vi "Live Capture Functional Stack4.64bit.vi"() -> ()   [LabVIEW 2014]
uses:
  subvis/Stack Track.ctl
  subvis/Stack_State.ctl
  Desktop/camtiff/ctiff.llb/__CTIFFNewFileAndStyleUINT16.vi
  Desktop/camtiff/ctiff.llb/__CTIFFAddNewPageUINT16.vi
  CameraControlTypeDef.ctl
panel:
  out "Image 2":u16[][](graph) caption="Image"
  in  "Slit Width / Lines 2":sgl=150.0
  out "Frame Index":i32
  in  "Temp":path=path "C:/temp.tmp"
  in  "Frames":i32=100
  in  "HardDisk Record":bool
  in  "Internal Line Interval":dbl
  in  "Slit Width / Lines":sgl=150.0
  in  "Camera Readout Mode":u16(ring)=12 items=["Full Frame"=1, "Slit Scanning"=12]
  in  "Readout Direction":sgl(ring)=1.0 items=["Forward"=1, "Backward"=2]
  in  "Trigger Mode":sgl(ring)=1.0 items=["Normal"=1, "Start "=6]
  in  "Trigger Source":sgl(ring)=2.0 items=["Internal"=1, "External"=2]
  out "State":T1=enum."Start Sequence"
  out "Image":u16[][](graph)
  out "Saving":bool
  in  "AutoIncrement":bool=TRUE
  in  "Path":path=path "C:/Users/spim/Desktop/Craig Cap/temp/a.tiff"
  in  "Frames":i32=100
  out "Frame Index":i32
  out "error out":errorcluster
  in  "stop":bool
  in  "Ram Record":bool
  out "Total Frames":i32
  out "Elapsed Time":u32
  out "Software FPS":dbl
  out "Camera FPS":dbl
  in  "H Offset":i32 min=0 max=0
  in  "H Width":i32 min=0 max=0
  out "SMD":dbl
  out "SHO":i32
  in  "V Offset":i32 min=0 max=0
  in  "V Width":i32 min=0 max=0
  in  "Binning":u16(ring) items=["1x1"=1, "2x2"=2, "4x4"=4]
  out "SHW":i32
  out "SVO":i32
  out "SVW":i32
  in  "Scan Mode":dbl min=0.0 max=0.0
  in  "Exposure":dbl min=0.0 max=0.0
  out "EXP":dbl
  out "Camera Model":string
  out "Camera Version":string
  out "Camera Serial":string
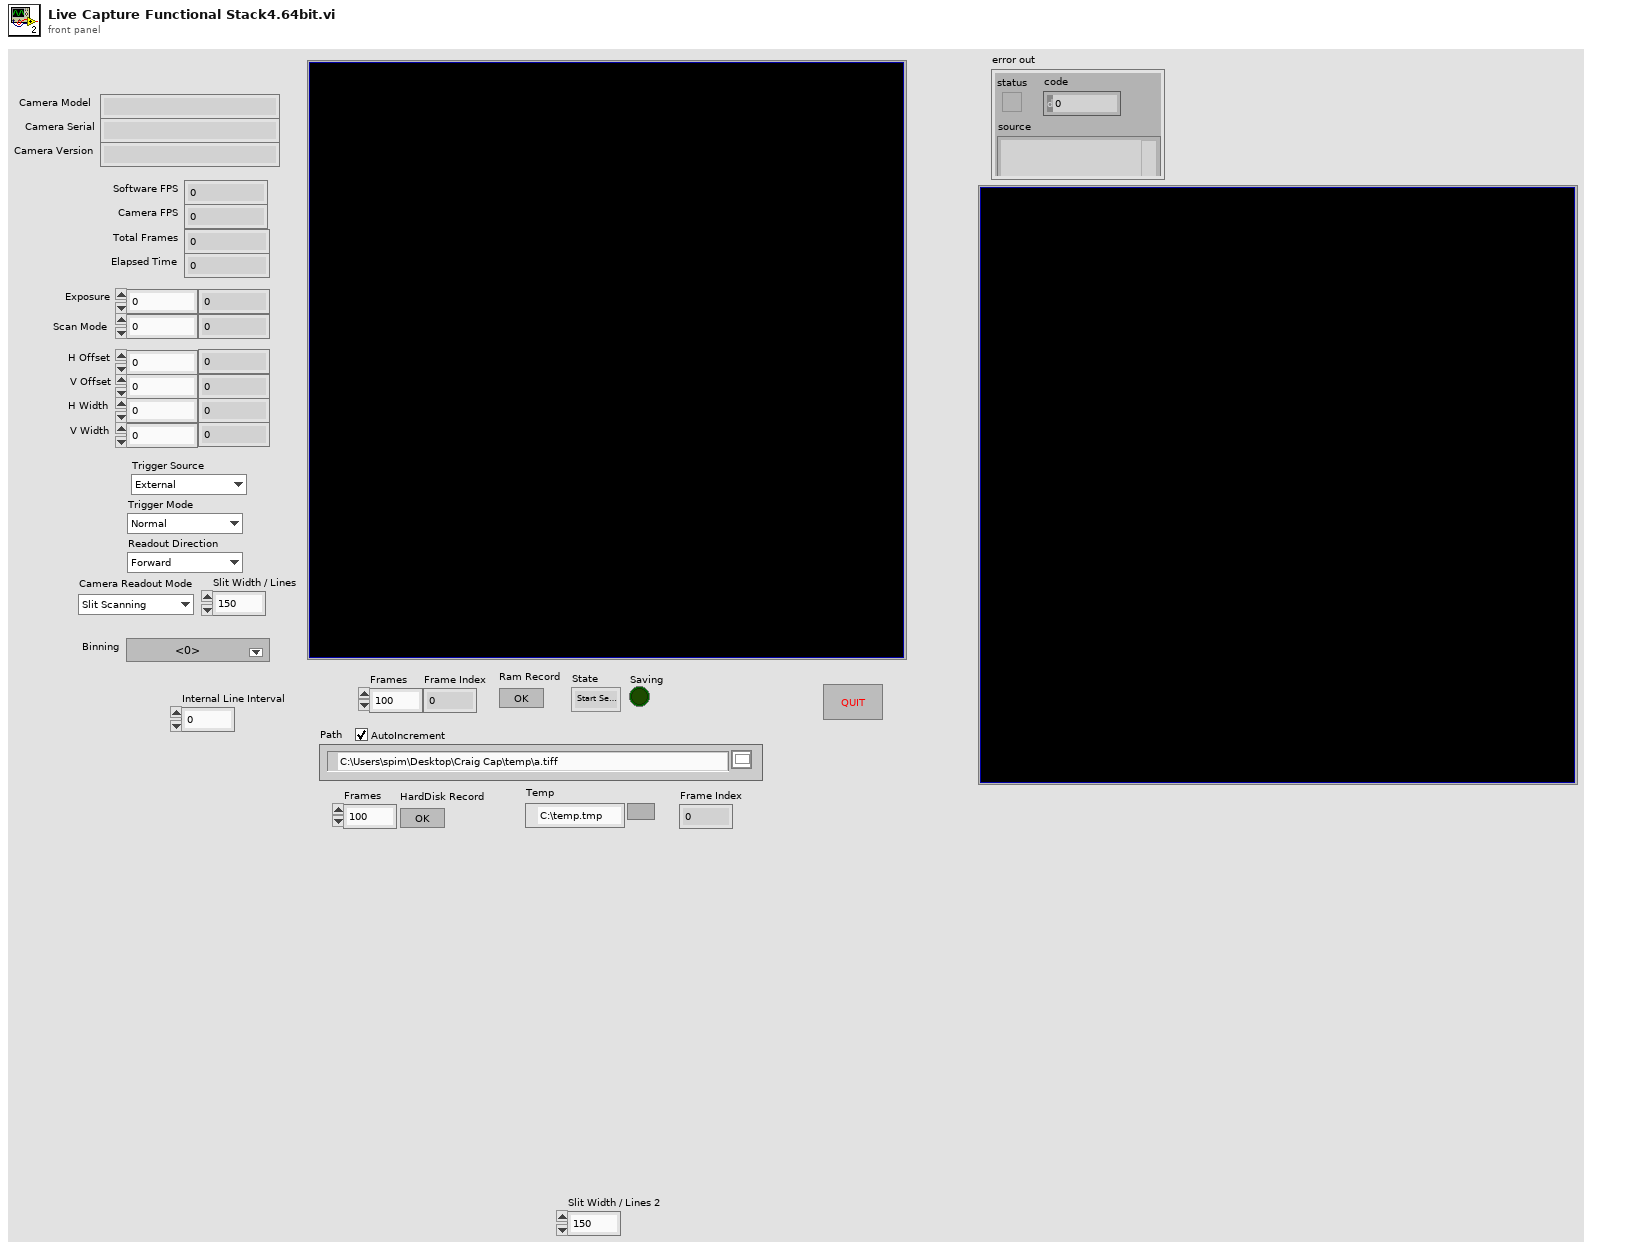
[diagram p1: front panel]
types:
  T1 = typedef "Stack Track.ctl" = enum16{"Idle", "Start Sequence", "Read Disk", "STOP", "Collecting", "End"}
  T2 = typedef "Stack_State.ctl" = cluster{"State":T1, "Stack Number":i32, "Image":u16[][]}
  T3 = typedef "CameraControlTypeDef.ctl" = enum16{"Ram Record", "HardDisk Record", "Disengage Update", "Update", "Idle"}
  T4 = enum8{"Enabled", "Disabled", "Disabled and Grayed Out"}
  T5 = cluster{"Model":string, "Camera ID":string, "Firmware":string}
  T6 = cluster{"Value":i32, "Minimum":i32, "Maximum":i32, "Increment":i32}
  T7 = cluster{"height":u32, "width":u32, "datatype":u32}
  T8 = cluster{"H Offset":i32, "V Offset":i32, "H Width":i32, "V Width":i32}
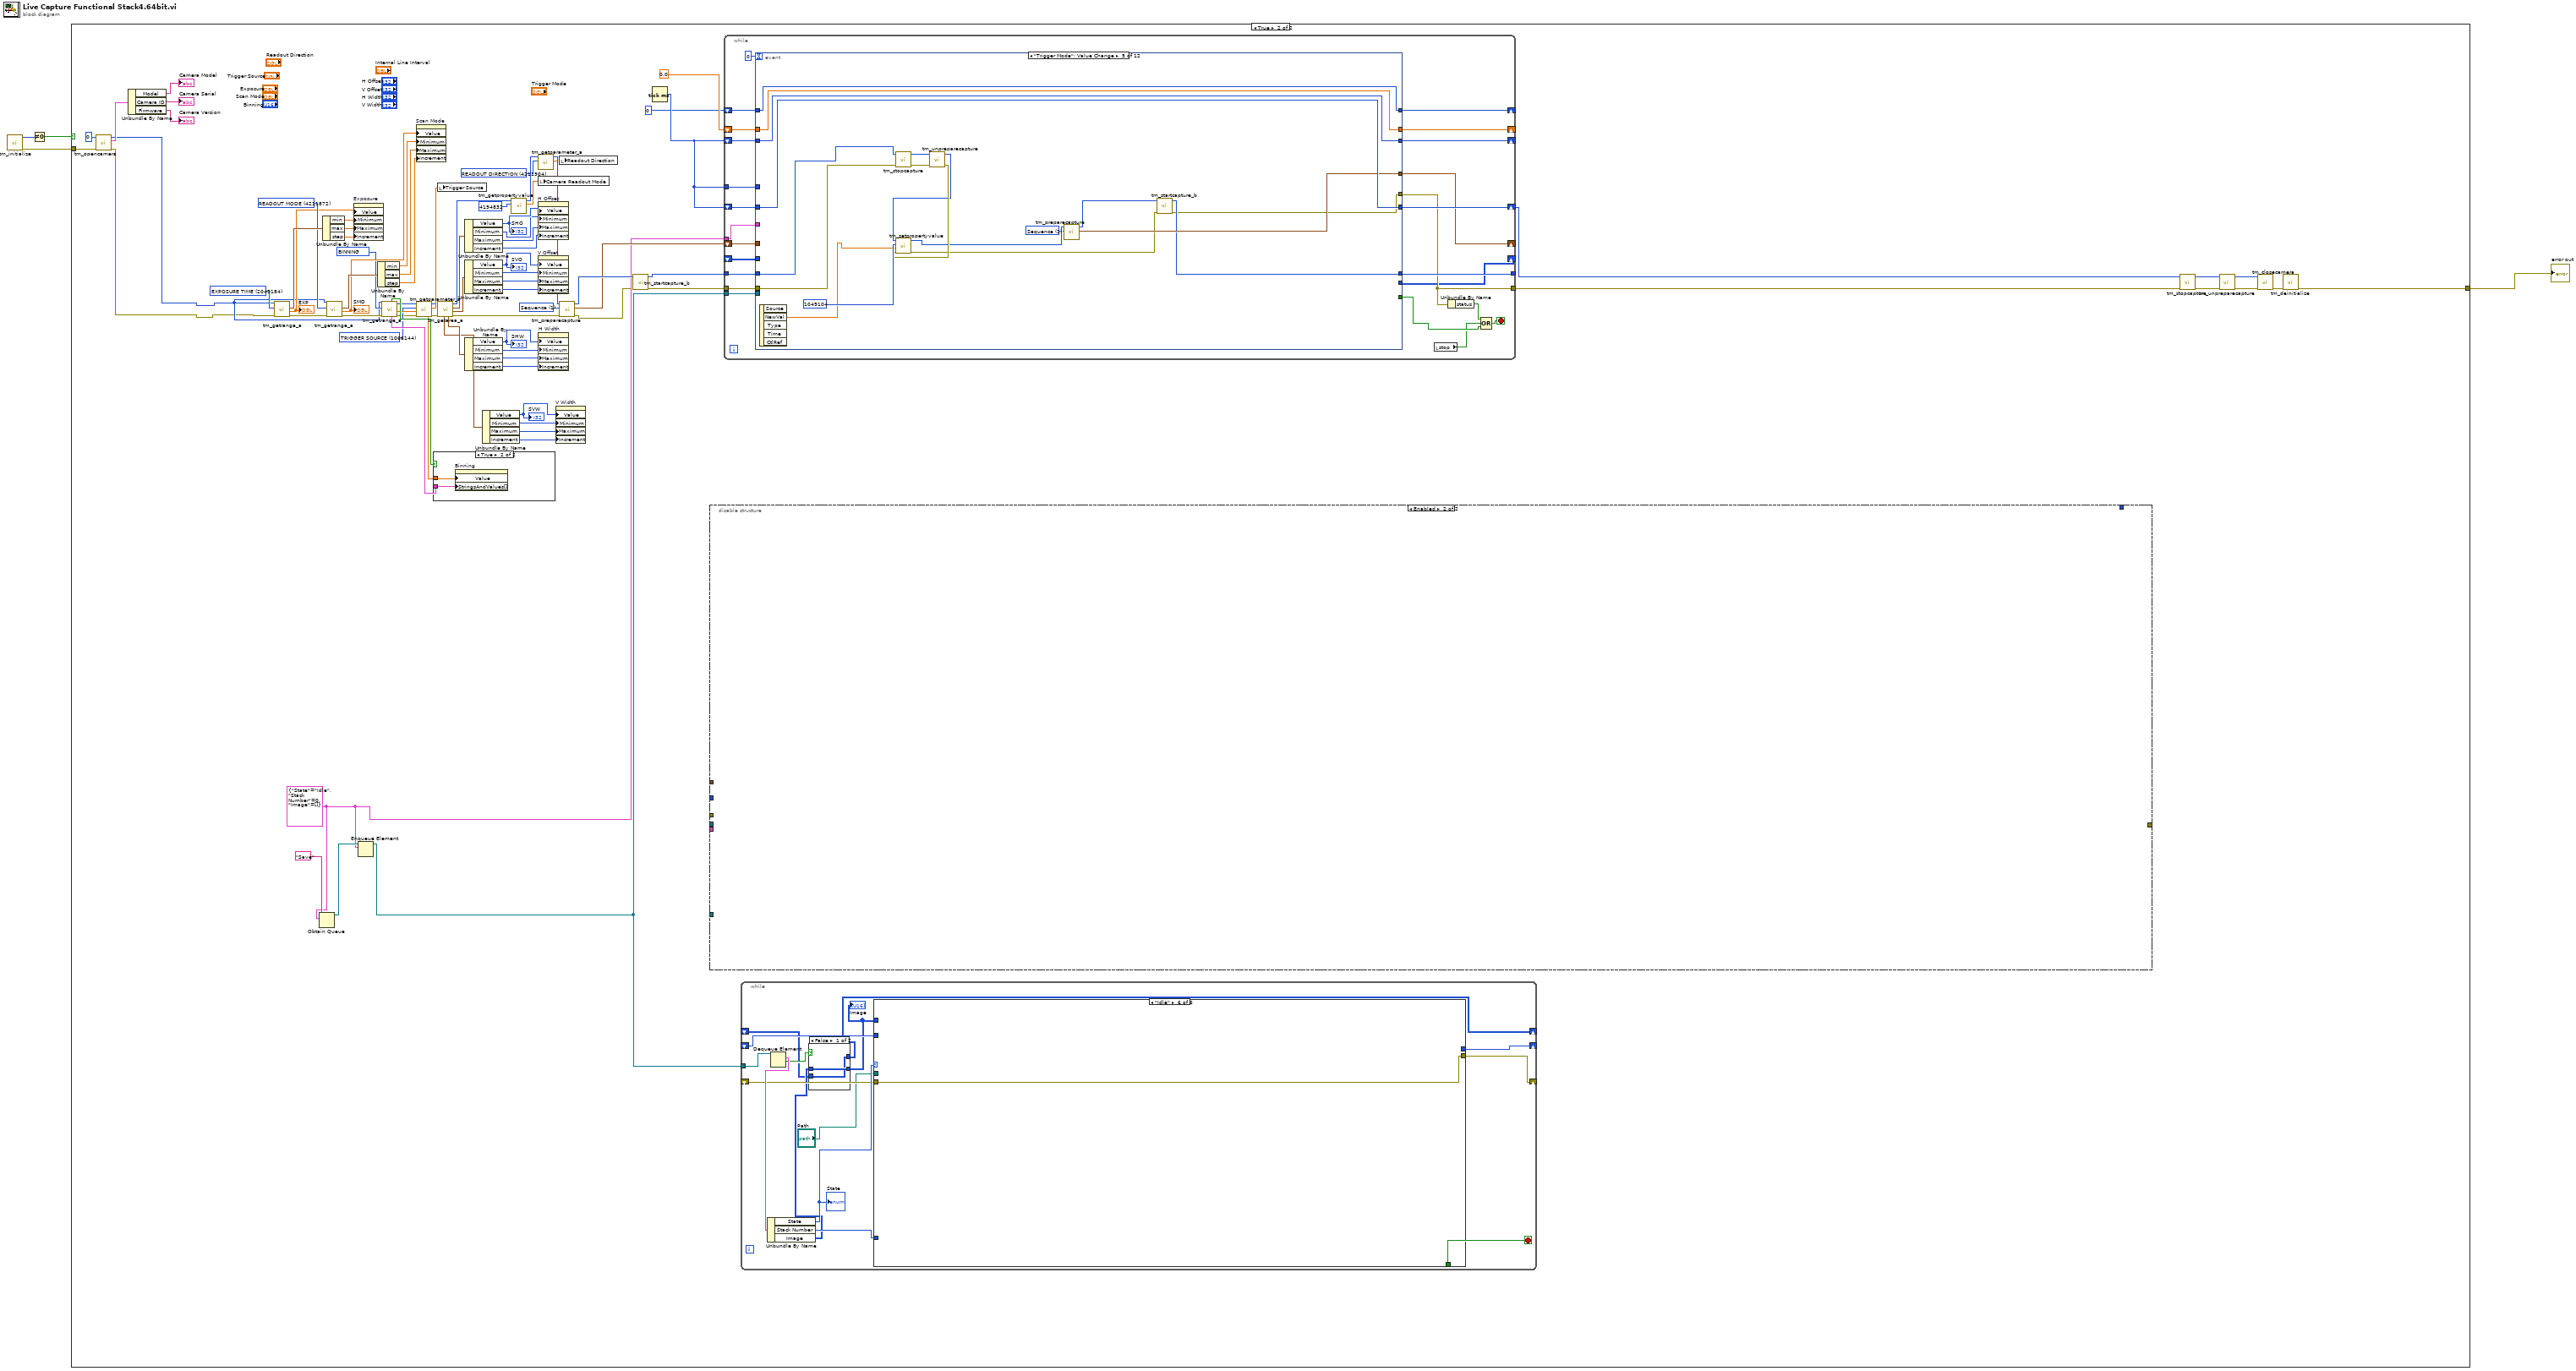
[diagram p0: block diagram]
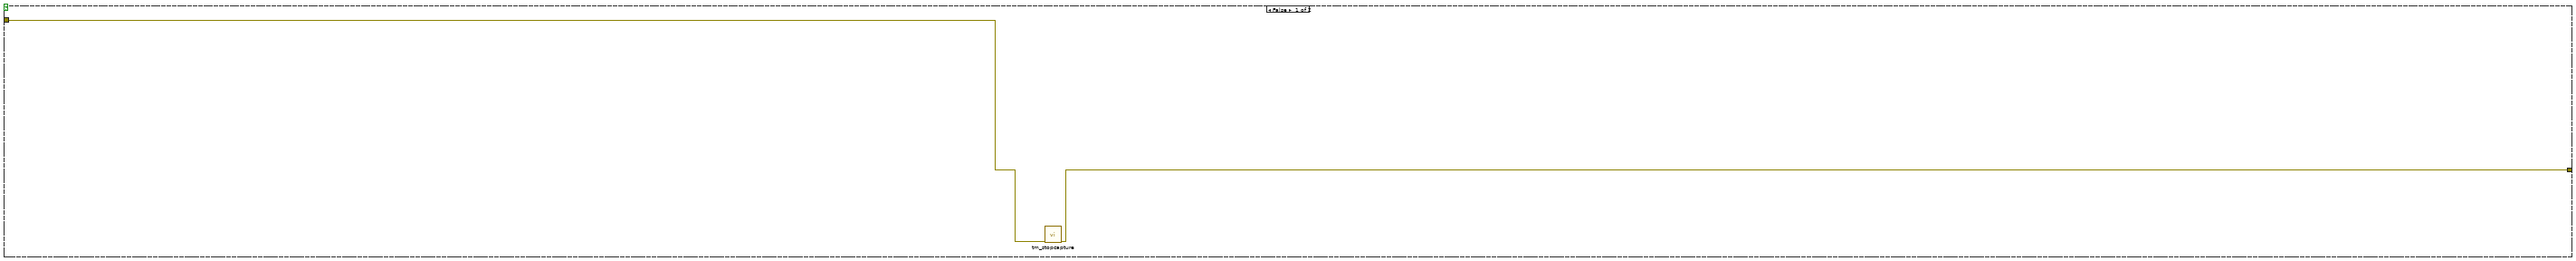
[diagram p2: hidden frame]
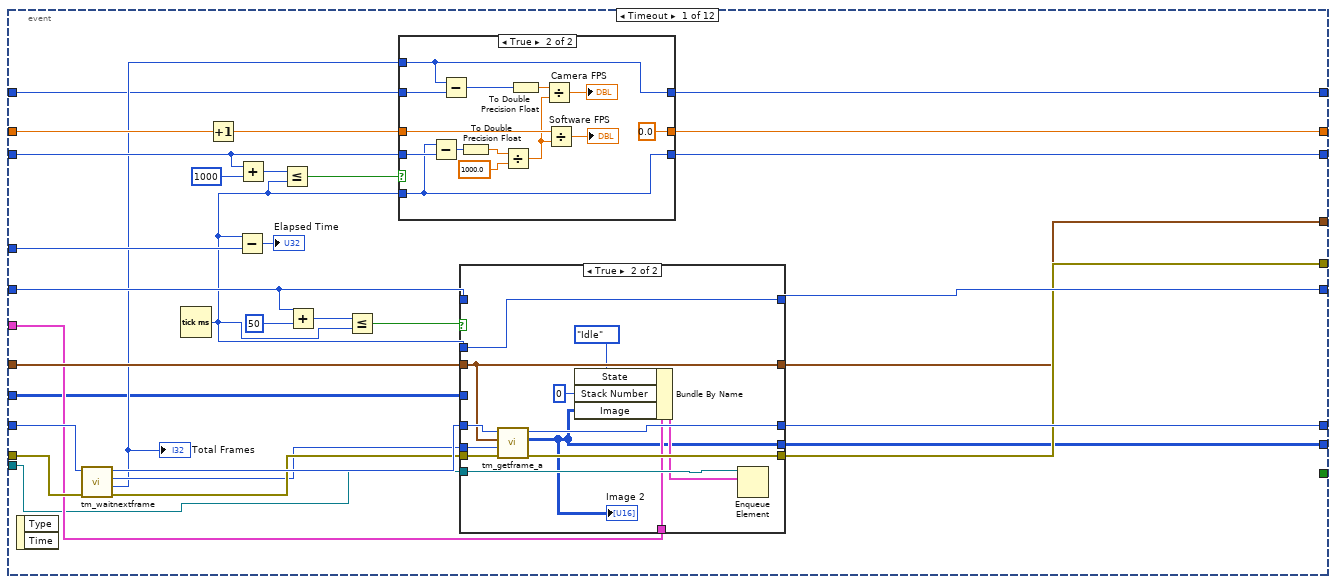
[diagram p3: hidden frame]
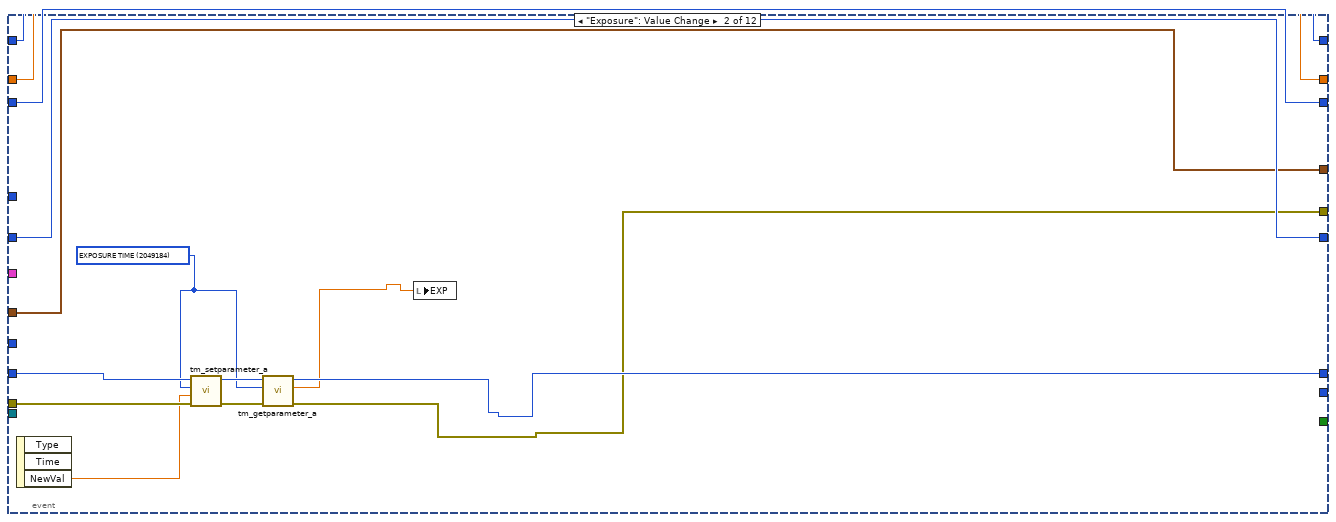
[diagram p6: hidden frame]
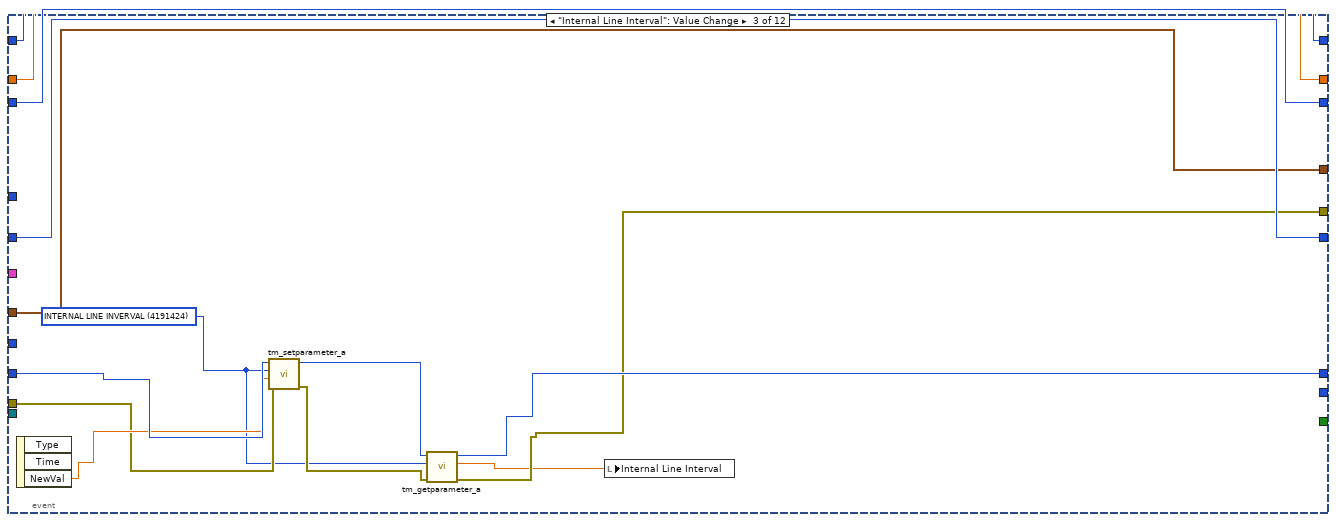
[diagram p7: hidden frame]
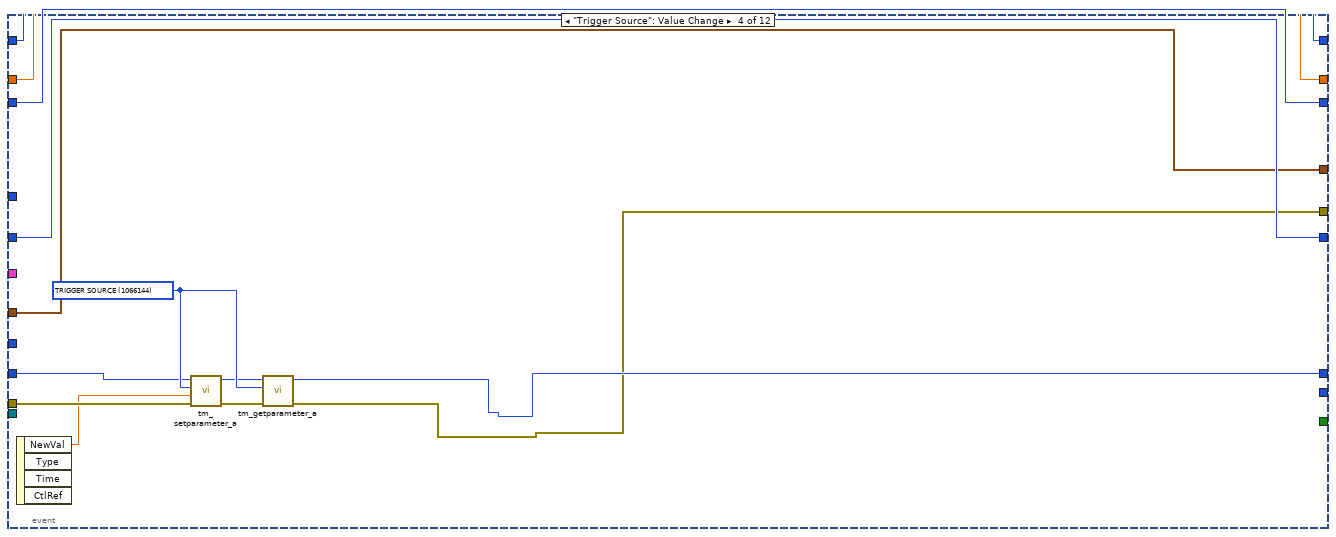
[diagram p8: hidden frame]
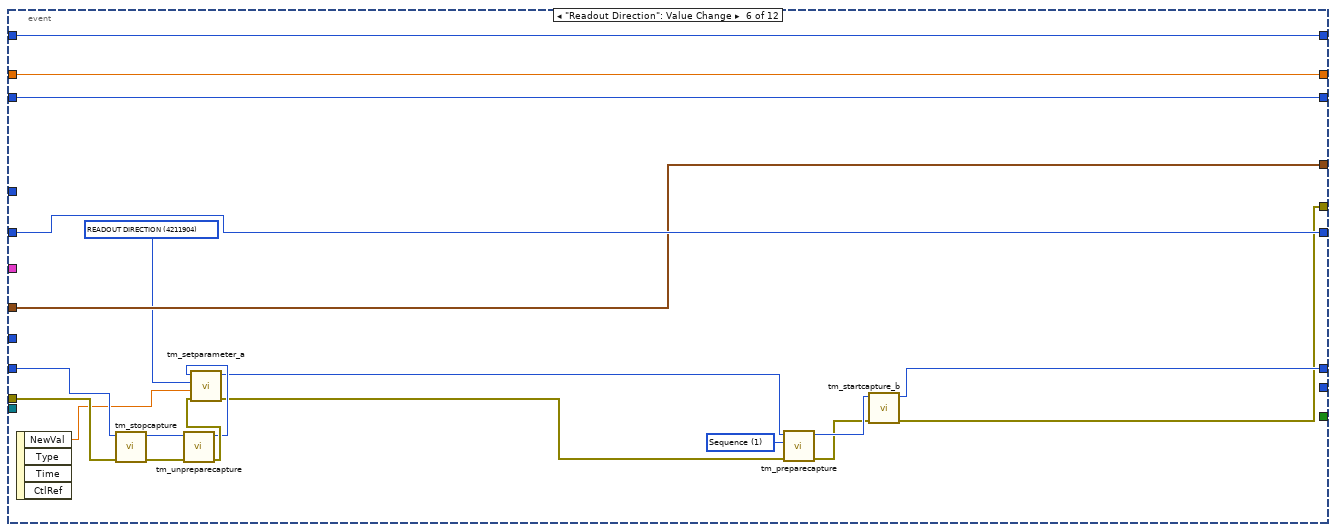
[diagram p9: hidden frame]
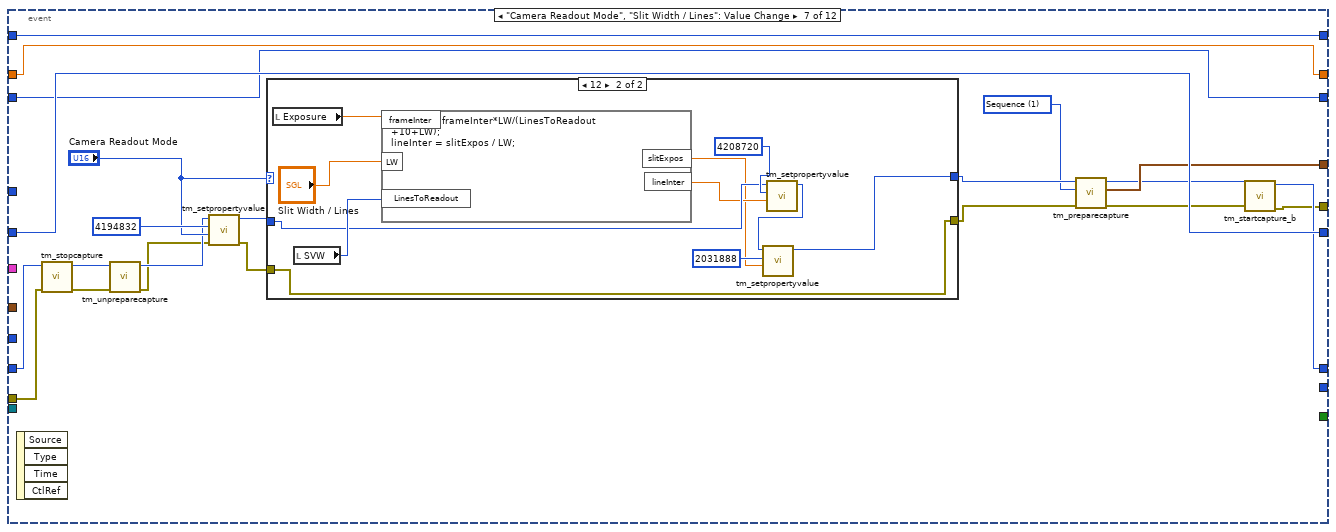
[diagram p10: hidden frame]
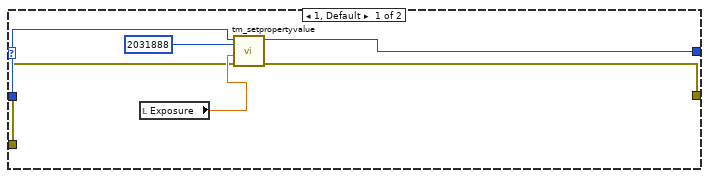
[diagram p11: hidden frame]
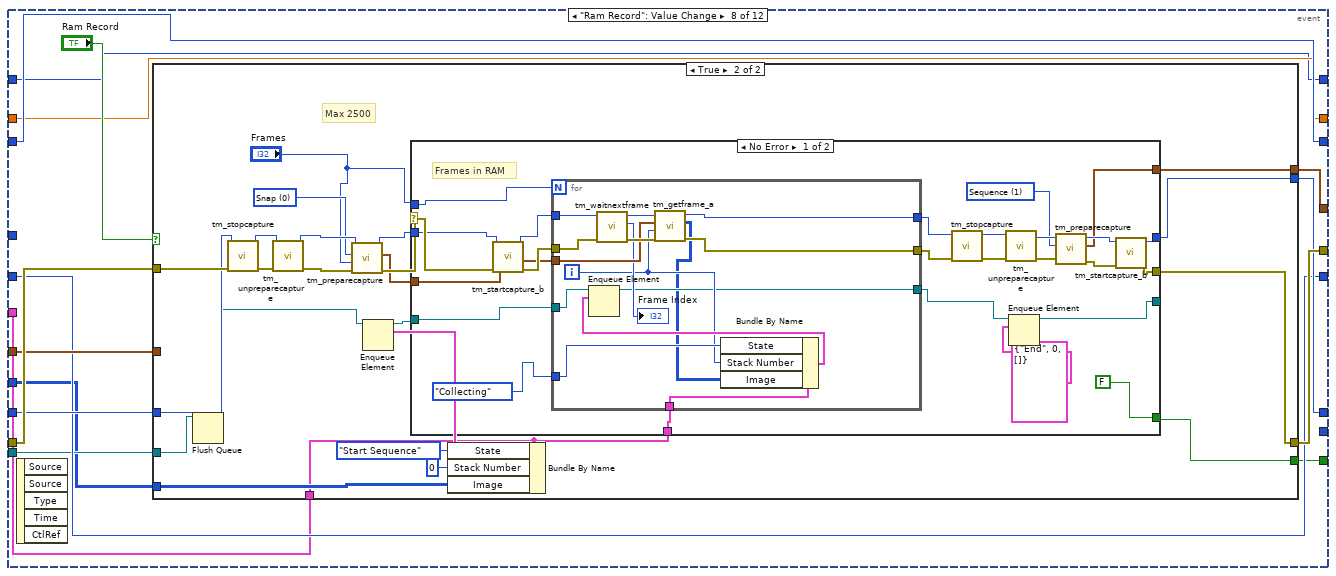
[diagram p12: hidden frame]
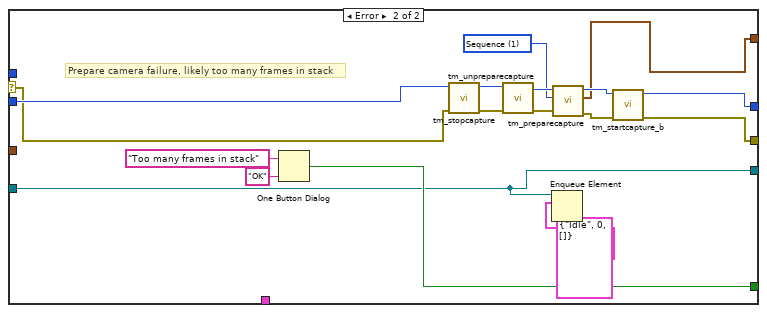
[diagram p14: hidden frame]
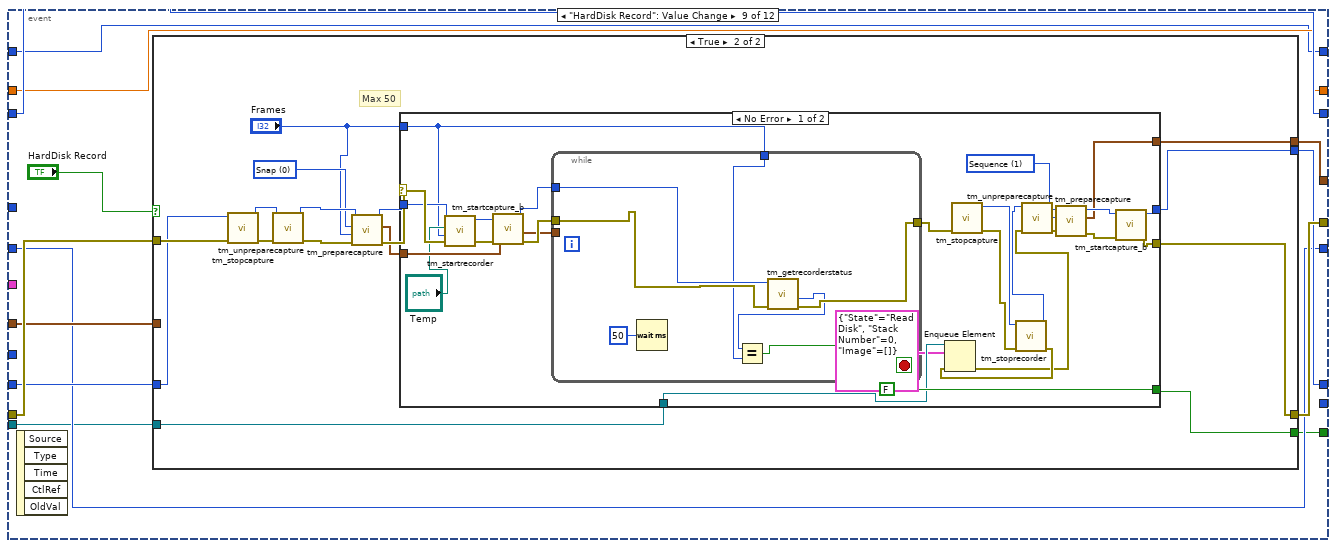
[diagram p15: hidden frame]
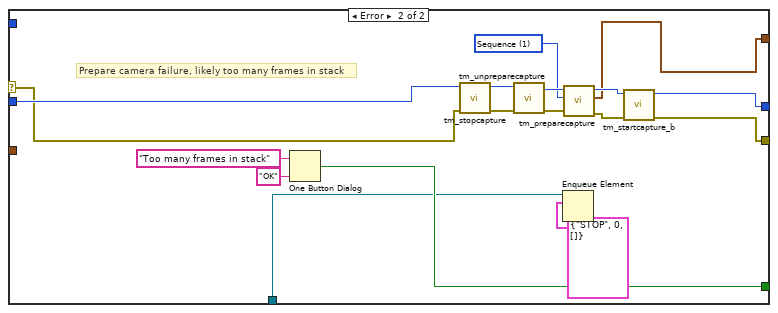
[diagram p17: hidden frame]
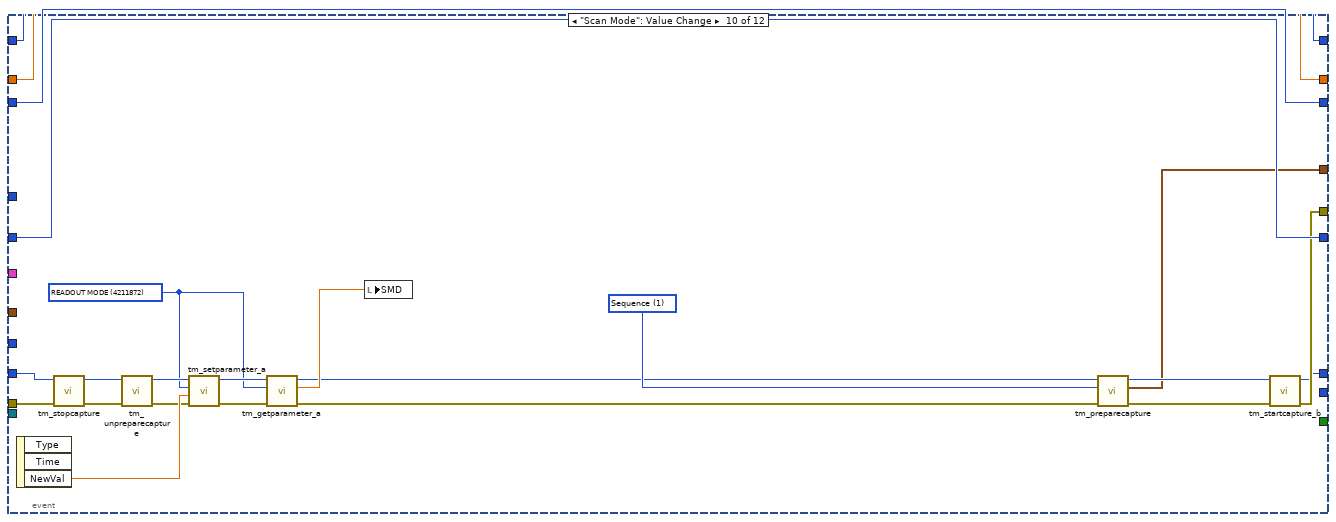
[diagram p18: hidden frame]
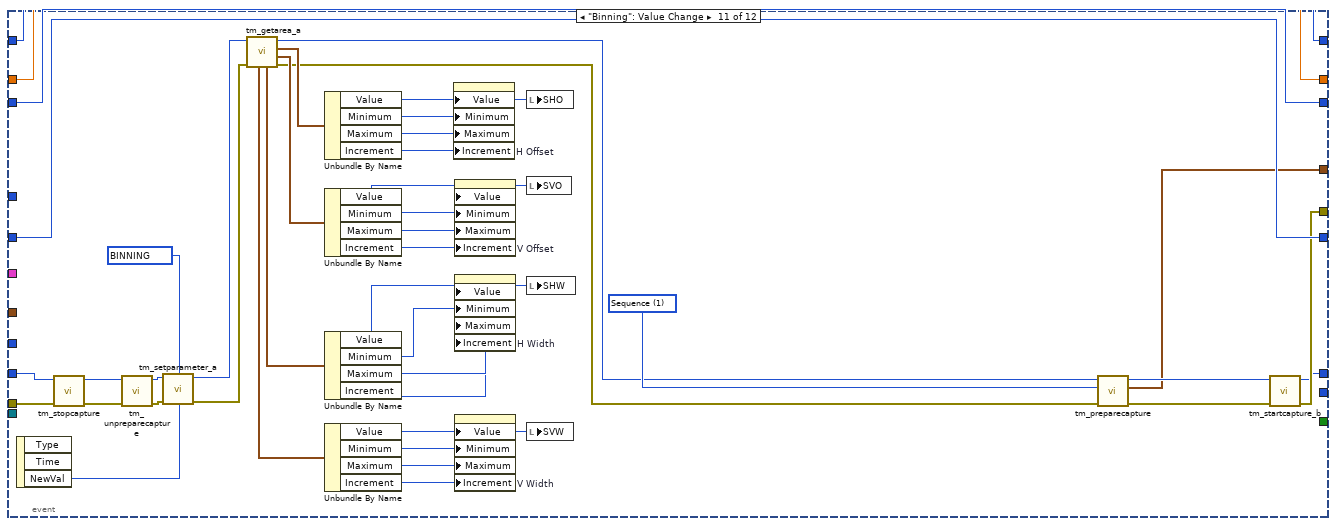
[diagram p19: hidden frame]
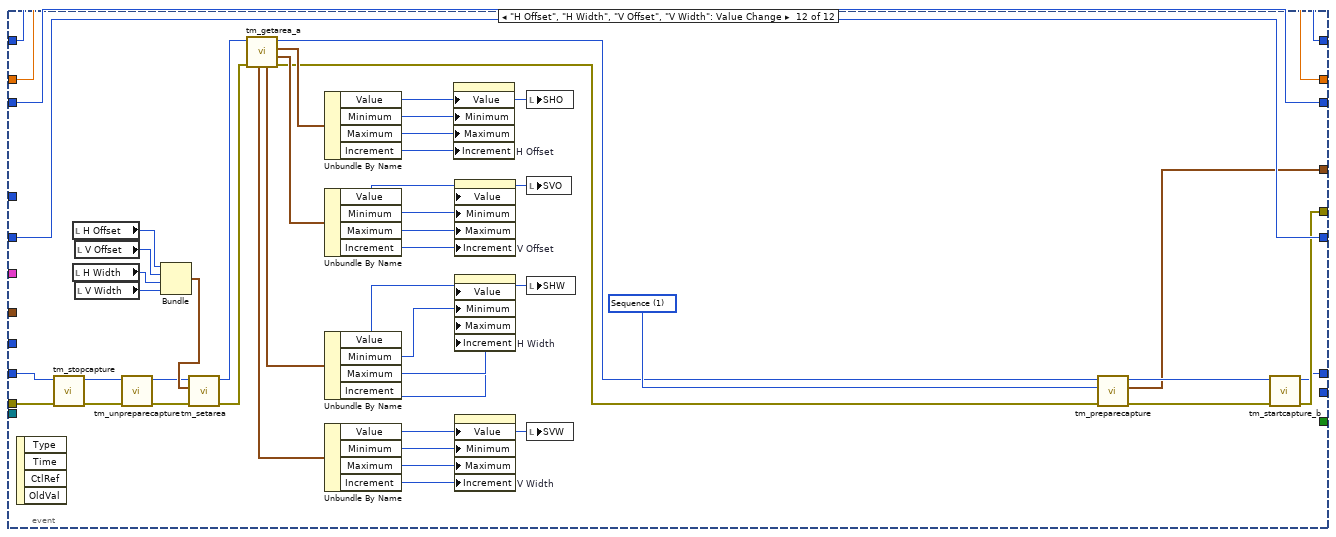
[diagram p20: hidden frame]
diagram:
  n1 = call <userlib>:"tm_initialize.vi"() -> ("error out"=w2:errorcluster, "Number Of Cameras"=w1:u32)  [unwired: 8 in, 2 out]
  n2 = Not Equal To 0?(x=w1) -> (x != 0?=w4:bool)
  n3 = case shown="True" w4 {
    tunnel: [w5 w84] -> w3
    tunnel: w2 -> [w6 w87]
    frame False {
      n4 = call <userlib>:"tm_stopcapture.vi"("error in (no error)"=w6) -> ("error out"=w5:errorcluster)  [unwired: 9 in, 1 out]
    }
    frame True {
      w19 = u32 4211904 items=["SENSOR MODE"=4212128, "CCD MODE"=4212384, "READOUT MODE"=4211872, "ACTIVE VIEW INDEX"=4343136, "BITS PER CHANNEL"=4342976, "IMAGE PIXEL TYPE"=4343296, "BINNING"=4215968, "EXPOSURE TIME"=2049184, "CONTRAST GAIN"=3163312, "CONTRAST OFFSET"=3163328, "LIGHT MODE"=2114720, "SENSITIVITY"=2114992, "PHOTON IMAGING MODE"=2115200, "HIGH DYNAMIC RANGE MODE"=3163360, "WHITE BALANCE"=3163568, "TEMPERATURE"=2115232, "TEMPERATURE TARGET"=2115264, "SENSOR COOLER FAN"=2115296, "LINEBUNDLE HEIGHT"=4212192, "MECHANICAL SHUTTER"=2115488, "BACK FOCUS POSITION"=8422304, "TRIGGER CONNECTOR"=1066432, "TRIGGER SOURCE"=1066144, "OUTPUT TRIGGER SOURCE"=1852576, "TRIGGER GLOBAL EXPOSURE"=2049680, "FIRST TRIGGER BEHAVIOR"=2049696, "CHANNEL SYNC"=1852352, "READOUT DIRECTION"=4211904, "PRE HSYNC COUNT"=1852704] ("Parameter")
      w29 = u32 1066144 items=["SENSOR MODE"=4212128, "CCD MODE"=4212384, "READOUT MODE"=4211872, "ACTIVE VIEW INDEX"=4343136, "BITS PER CHANNEL"=4342976, "IMAGE PIXEL TYPE"=4343296, "BINNING"=4215968, "EXPOSURE TIME"=2049184, "CONTRAST GAIN"=3163312, "CONTRAST OFFSET"=3163328, "LIGHT MODE"=2114720, "SENSITIVITY"=2114992, "PHOTON IMAGING MODE"=2115200, "HIGH DYNAMIC RANGE MODE"=3163360, "WHITE BALANCE"=3163568, "TEMPERATURE"=2115232, "TEMPERATURE TARGET"=2115264, "SENSOR COOLER FAN"=2115296, "LINEBUNDLE HEIGHT"=4212192, "MECHANICAL SHUTTER"=2115488, "BACK FOCUS POSITION"=8422304, "TRIGGER CONNECTOR"=1066432, "TRIGGER SOURCE"=1066144, "OUTPUT TRIGGER SOURCE"=1852576, "TRIGGER GLOBAL EXPOSURE"=2049680, "FIRST TRIGGER BEHAVIOR"=2049696, "CHANNEL SYNC"=1852352, "READOUT DIRECTION"=4211904, "PRE HSYNC COUNT"=1852704] ("Parameter")
      w12 = T2 {"State"=enum."Idle", "Stack Number"=0, "Image"=[]} ("input cluster")
      w34 = u32 2049184 items=["BINNING"=4215968, "BITS PER CHANNEL"=4342976, "ACTIVE VIEW INDEX"=4343136, "CCD MODE"=4212384, "SENSOR MODE"=4212128, "READOUT MODE"=4211872, "EXPOSURE TIME"=2049184, "CONTRAST GAIN"=3163312, "CONTRAST OFFSET"=3163328, "LIGHT MODE"=2114720, "SENSITIVITY"=2114992, "WHITE BALANCE"=3163568, "PHOTON IMAGING MODE"=2115200, "HIGH DYNAMIC RANGE MODE"=3163360, "TRIGGER SOURCE"=1066144, "TRIGGER ACTIVE"=1066160, "TRIGGER MODE"=1066400, "TRIGGER POLARITY"=1066416, "TRIGGER GLOBAL EXPOSURE"=2049680, "FIRST TRIGGER BEHAVIOR"=2049696, "TRIGGER TIMES"=1066448, "OUTPUT TRIGGER POLARITY"=1852592, "OUTPUT TRIGGER DELAY"=1852624, "OUTPUT TRIGGER PERIOD"=1852640, "TEMPERATURE"=2115232, "TEMPERATURE TARGET"=2115264, "SENSOR COOLER FAN"=2115296, "MECHANICAL SHUTTER"=2115488, "BACK FOCUS POSITION"=8422304, "FRAMEBUNDLE MODE"=4346784, "FRAMEBUNDLE NUMBER"=4346800, "LINEBUNDLE HEIGHT"=4212192, "TRIGGER CONNECTOR"=1066432, "IMAGE PIXEL TYPE"=4343296, "OUTPUT TRIGGER KIND"=1852656, "READOUT DIRECTION"=4211904, "CHANNEL SYNC"=1852352] ("Parameter")
      w35 = u32 4211872 items=["BINNING"=4215968, "BITS PER CHANNEL"=4342976, "ACTIVE VIEW INDEX"=4343136, "CCD MODE"=4212384, "SENSOR MODE"=4212128, "READOUT MODE"=4211872, "EXPOSURE TIME"=2049184, "CONTRAST GAIN"=3163312, "CONTRAST OFFSET"=3163328, "LIGHT MODE"=2114720, "SENSITIVITY"=2114992, "WHITE BALANCE"=3163568, "PHOTON IMAGING MODE"=2115200, "HIGH DYNAMIC RANGE MODE"=3163360, "TRIGGER SOURCE"=1066144, "TRIGGER ACTIVE"=1066160, "TRIGGER MODE"=1066400, "TRIGGER POLARITY"=1066416, "TRIGGER GLOBAL EXPOSURE"=2049680, "FIRST TRIGGER BEHAVIOR"=2049696, "TRIGGER TIMES"=1066448, "OUTPUT TRIGGER POLARITY"=1852592, "OUTPUT TRIGGER DELAY"=1852624, "OUTPUT TRIGGER PERIOD"=1852640, "TEMPERATURE"=2115232, "TEMPERATURE TARGET"=2115264, "SENSOR COOLER FAN"=2115296, "MECHANICAL SHUTTER"=2115488, "BACK FOCUS POSITION"=8422304, "FRAMEBUNDLE MODE"=4346784, "FRAMEBUNDLE NUMBER"=4346800, "LINEBUNDLE HEIGHT"=4212192, "TRIGGER CONNECTOR"=1066432, "IMAGE PIXEL TYPE"=4343296, "OUTPUT TRIGGER KIND"=1852656, "READOUT DIRECTION"=4211904, "CHANNEL SYNC"=1852352] ("Parameter")
      w36 = u32 4215968 items=["BINNING"=4215968, "BITS PER CHANNEL"=4342976, "ACTIVE VIEW INDEX"=4343136, "CCD MODE"=4212384, "SENSOR MODE"=4212128, "READOUT MODE"=4211872, "EXPOSURE TIME"=2049184, "CONTRAST GAIN"=3163312, "CONTRAST OFFSET"=3163328, "LIGHT MODE"=2114720, "SENSITIVITY"=2114992, "WHITE BALANCE"=3163568, "PHOTON IMAGING MODE"=2115200, "HIGH DYNAMIC RANGE MODE"=3163360, "TRIGGER SOURCE"=1066144, "TRIGGER ACTIVE"=1066160, "TRIGGER MODE"=1066400, "TRIGGER POLARITY"=1066416, "TRIGGER GLOBAL EXPOSURE"=2049680, "FIRST TRIGGER BEHAVIOR"=2049696, "TRIGGER TIMES"=1066448, "OUTPUT TRIGGER POLARITY"=1852592, "OUTPUT TRIGGER DELAY"=1852624, "OUTPUT TRIGGER PERIOD"=1852640, "TEMPERATURE"=2115232, "TEMPERATURE TARGET"=2115264, "SENSOR COOLER FAN"=2115296, "MECHANICAL SHUTTER"=2115488, "BACK FOCUS POSITION"=8422304, "FRAMEBUNDLE MODE"=4346784, "FRAMEBUNDLE NUMBER"=4346800, "LINEBUNDLE HEIGHT"=4212192, "TRIGGER CONNECTOR"=1066432, "IMAGE PIXEL TYPE"=4343296, "OUTPUT TRIGGER KIND"=1852656, "READOUT DIRECTION"=4211904, "CHANNEL SYNC"=1852352] ("Parameter")
      w82 = 1 items=["Snap", "Sequence"] ("Capture mode")
      n5 = call <userlib>:"tm_opencamera.vi"("error in (no error)"=w87, "Camera Index"=u32 0) -> ("error out"=w7:errorcluster, "Camera Details"=w48:T5, "Handle out"=w8:u32)  [unwired: 7 in]
      n6 = Unbundle By Name(w48) -> ("Model"=→"Camera Model":string, "Camera ID"=→"Camera Serial":string, "Firmware"=→"Camera Version":string)
      n7 = call <userlib>:"tm_getrange_a.vi"("error in (no error)"=w7, "Parameter"=w34, "Handle in"=w8) -> ("error out"=w43:errorcluster, "default"=w32:dbl, "Range"=w44:cluster{"min":dbl, "max":dbl, "step":dbl})  [unwired: 2 in, 4 out]
      "EXP" <- w32
      n8 = Obtain Queue(name (unnamed)="Save", element data type=w12) -> (queue out=w16:refnum<queue>)  [unwired: 3 in, 2 out]
      n9 = Unbundle By Name(w44) -> ("min"=w79:dbl, "max"=w78:dbl, "step"=w77:dbl)
      n10 = call <userlib>:"tm_getrange_a.vi"("error in (no error)"=w43, "Parameter"=w35, "Handle in"=w8) -> ("error out"=w40:errorcluster, "default"=w41:dbl, "Range"=w42:cluster{"min":dbl, "max":dbl, "step":dbl})  [unwired: 2 in, 4 out]
      "SMD" <- w41
      n11 = property on="Exposure" class="DigNum (strict)"("Value"=w32, "Minimum"=w79, "Maximum"=w78, "Increment"=w77) -> ()  [unwired: 2 in, 2 out]
      n12 = Enqueue Element(queue=w16, element=w12) -> (queue out=w15:refnum<queue>)  [unwired: 2 in, 2 out]
      n13 = Unbundle By Name(w42) -> ("min"=w76:dbl, "max"=w75:dbl, "step"=w74:dbl)
      n14 = call <userlib>:"tm_getrange_a.vi"("error in (no error)"=w40, "Parameter"=w36, "Handle in"=w8) -> ("error out"=w26:errorcluster, "default"=w38:dbl, "Handle out"=w28:u32, "Value Names"=w37:cluster{"Name":string, "Value":dbl}[], "Writable"=w39:bool)  [unwired: 2 in, 2 out]
      n15 = property on="Scan Mode" class="DigNum (strict)"("Value"=w41, "Minimum"=w76, "Maximum"=w75, "Increment"=w74) -> ()  [unwired: 2 in, 2 out]
      n16 = call <userlib>:"tm_getparameter_a.vi"("error in (no error)"=w26, "Parameter"=w29, "Handle in"=w28) -> ("error out"=w25:errorcluster, "Value out"=w30:dbl, "Handle out"=w27:u32)  [unwired: 6 in]
      n17 = case shown="True" w39 {
        tunnel: w37 -> [_ w833]
        tunnel: w38 -> [_ w832]
        frame False {
        }
        frame True {
          n18 = property on="Binning" class="Ring (strict)"("Value"=w832, "StringsAndValues[]"=w833) -> ()  [unwired: 2 in, 2 out]
        }
      }
      n19 = local write "Trigger Source"(w30) -> ()
      n20 = call <userlib>:"tm_getarea_a.vi"("error in (no error)"=w25, "Handle in"=w27) -> ("error out"=w31:errorcluster, "V Offset"=w73:T6, "H Offset"=w54:T6, "Handle out"=w22:u32, "H Width"=w72:T6, "V Width"=w71:T6)  [unwired: 4 in]
      n21 = Unbundle By Name(w54) -> ("Value"=w53:i32, "Minimum"=w52:i32, "Maximum"=w51:i32, "Increment"=w50:i32)
      "SHO" <- w53
      n22 = Unbundle By Name(w73) -> ("Value"=w61:i32, "Minimum"=w70:i32, "Maximum"=w69:i32, "Increment"=w68:i32)
      "SVO" <- w61
      n23 = Unbundle By Name(w72) -> ("Value"=w60:i32, "Minimum"=w67:i32, "Maximum"=w66:i32, "Increment"=w65:i32)
      "SHW" <- w60
      n24 = Unbundle By Name(w71) -> ("Value"=w59:i32, "Minimum"=w64:i32, "Maximum"=w63:i32, "Increment"=w62:i32)
      "SVW" <- w59
      n25 = call <userlib>:"tm_getpropertyvalue.vi"("Property ID"=u32 4194832, "Handle in"=w22) -> ("Value in"=w23:sgl, "Handle out"=w21:u32)  [unwired: 7 in, 1 out]
      n26 = call <userlib>:"tm_getparameter_a.vi"("Parameter"=w19, "Handle in"=w21) -> ("Value out"=w18:dbl, "Handle out"=w20:u32)  [unwired: 7 in, 1 out]
      n27 = local write "Camera Readout Mode"(w23) -> ()
      n28 = property on="H Offset" class="DigNum (strict)"("Value"=w53, "Minimum"=w52, "Maximum"=w51, "Increment"=w50) -> ()  [unwired: 2 in, 2 out]
      n29 = property on="V Offset" class="DigNum (strict)"("Value"=w61, "Minimum"=w70, "Maximum"=w69, "Increment"=w68) -> ()  [unwired: 2 in, 2 out]
      n30 = property on="H Width" class="DigNum (strict)"("Value"=w60, "Minimum"=w67, "Maximum"=w66, "Increment"=w65) -> ()  [unwired: 2 in, 2 out]
      n31 = property on="V Width" class="DigNum (strict)"("Value"=w59, "Minimum"=w64, "Maximum"=w63, "Increment"=w62) -> ()  [unwired: 2 in, 2 out]
      n32 = local write "Readout Direction"(w18) -> ()
      n33 = call <userlib>:"tm_preparecapture.vi"("error in (no error)"=w31, "Capture mode"=w82, "Handle in"=w20) -> ("error out"=w11:errorcluster, "Buffer Info"=w13:T7, "Handle out"=w17:u32)  [unwired: 5 in, 1 out]
      n34 = call <userlib>:"tm_startcapture_b.vi"("error in (no error)"=w11, "Handle in"=w17) -> ("error out"=w81:errorcluster, "Handle out"=w14:u32)  [unwired: 8 in]
      n35 = Tick Count (ms)() -> (millisecond timer value=w80:u32)
      n36 = disable-structure shown="Enabled" {
        disable-tunnel: _ -> [w594 _]
        disable-tunnel: _ -> [w593 _]
        disable-tunnel: _ -> [w592 _]
        disable-tunnel: _ -> [w591 _]
        disable-tunnel: _ -> [w590 _]
        disable-tunnel: [w589 _] -> _
        disable-tunnel: [w588 _] -> _
        disable-tunnel: _ -> [w587 _]
        frame Disabled {
          n37 = while {
            tunnel: w594 -> [w609]
            tunnel: w587 -> [w612]
            tunnel: w591 -> [w608]
            shift-right: [w607] -> _
            shift-left: w592 -> [w610]
            shift-right: [w606] -> w588
            shift-left: w593 -> [w611]
            tunnel: w590 -> [w605]
            tunnel: [w604] -> w589
            stop <- w599 stop-if-true
            n38 = Dequeue Element(queue=w612, timeout in ms (-1)=1) -> (element=w600:T3, timed out?=w602:bool)  [unwired: 1 in, 2 out]
            n39 = case shown="True" w602 {
              tunnel: [w613 CameraControlTypeDef."Idle" ("Enum")] -> w601
              tunnel: w600 -> [w613 _]
              frame False {
              }
              frame True {
              }
            }
            n40 = case shown="\"Idle\", Default" w601 {
              selector: w601 -> [_ _ w693 _ _]
              tunnel: w611 -> [w617 w618 _ w731 w748]
              tunnel: w610 -> [w616 w620 _ w716 w740]
              tunnel: w609 -> [_ _ _ _ w746]
              tunnel: w608 -> [_ _ _ _ w745]
              tunnel: [w616 w620 w631 w716 w740] -> w607
              tunnel: [w617 w618 w621 w717 w739] -> w606
              tunnel: w605 -> [w615 w619 w690 w730 w736]
              tunnel: [w615 w619 w630 w715 w738] -> w604
              frame "Ram Record" {
              }
              frame "HardDisk Record" {
              }
              frame "Disengage Update" {
                w634 = 1 items=["Snap", "Sequence"] ("Capture mode")
                w637 = u32 4215968 items=["BINNING"=4215968, "BITS PER CHANNEL"=2, "ACTIVE VIEW INDEX"=3, "CCD MODE"=4, "SENSOR MODE"=5, "READOUT MODE"=6, "EXPOSURE TIME"=7, "CONTRAST GAIN"=8, "CONTRAST OFFSET"=9, "LIGHT MODE"=10, "SENSITIVITY"=11, "WHITE BALANCE"=12, "PHOTON IMAGING MODE"=13, "HIGH DYNAMIC RANGE MODE"=14, "TRIGGER SOURCE"=15, "TRIGGER ACTIVE"=16, "TRIGGER MODE"=17, "TRIGGER POLARITY"=18, "TRIGGER GLOBAL EXPOSURE"=19, "FIRST TRIGGER BEHAVIOR"=20, "TRIGGER TIMES"=21, "OUTPUT TRIGGER POLARITY"=22, "OUTPUT TRIGGER DELAY"=23, "OUTPUT TRIGGER PERIOD"=24, "TEMPERATURE"=25, "TEMPERATURE TARGET"=26, "SENSOR COOLER FAN"=27, "MECHANICAL SHUTTER"=28, "BACK FOCUS POSITION"=29, "FRAMEBUNDLE MODE"=30, "FRAMEBUNDLE NUMBER"=31, "LINEBUNDLE HEIGHT"=32, "TRIGGER CONNECTOR"=33, "IMAGE PIXEL TYPE"=34, "OUTPUT TRIGGER KIND"=35, "READOUT DIRECTION"=36, "CHANNEL SYNC"=37] ("Parameter")
                w664 = u32 4211872 items=["SENSOR MODE"=4212128, "CCD MODE"=4212384, "READOUT MODE"=4211872, "ACTIVE VIEW INDEX"=4343136, "BITS PER CHANNEL"=4342976, "IMAGE PIXEL TYPE"=4343296, "BINNING"=4215968, "EXPOSURE TIME"=2049184, "CONTRAST GAIN"=3163312, "CONTRAST OFFSET"=3163328, "LIGHT MODE"=2114720, "SENSITIVITY"=2114992, "PHOTON IMAGING MODE"=2115200, "HIGH DYNAMIC RANGE MODE"=3163360, "WHITE BALANCE"=3163568, "TEMPERATURE"=2115232, "TEMPERATURE TARGET"=2115264, "SENSOR COOLER FAN"=2115296, "LINEBUNDLE HEIGHT"=4212192, "MECHANICAL SHUTTER"=2115488, "BACK FOCUS POSITION"=8422304, "TRIGGER CONNECTOR"=1066432, "TRIGGER SOURCE"=1066144, "OUTPUT TRIGGER SOURCE"=1852576, "TRIGGER GLOBAL EXPOSURE"=2049680, "FIRST TRIGGER BEHAVIOR"=2049696, "CHANNEL SYNC"=1852352, "READOUT DIRECTION"=4211904, "PRE HSYNC COUNT"=1852704] ("Parameter")
                w677 = u32 4211904 items=["SENSOR MODE"=4212128, "CCD MODE"=4212384, "READOUT MODE"=4211872, "ACTIVE VIEW INDEX"=4343136, "BITS PER CHANNEL"=4342976, "IMAGE PIXEL TYPE"=4343296, "BINNING"=4215968, "EXPOSURE TIME"=2049184, "CONTRAST GAIN"=3163312, "CONTRAST OFFSET"=3163328, "LIGHT MODE"=2114720, "SENSITIVITY"=2114992, "PHOTON IMAGING MODE"=2115200, "HIGH DYNAMIC RANGE MODE"=3163360, "WHITE BALANCE"=3163568, "TEMPERATURE"=2115232, "TEMPERATURE TARGET"=2115264, "SENSOR COOLER FAN"=2115296, "LINEBUNDLE HEIGHT"=4212192, "MECHANICAL SHUTTER"=2115488, "BACK FOCUS POSITION"=8422304, "TRIGGER CONNECTOR"=1066432, "TRIGGER SOURCE"=1066144, "OUTPUT TRIGGER SOURCE"=1852576, "TRIGGER GLOBAL EXPOSURE"=2049680, "FIRST TRIGGER BEHAVIOR"=2049696, "CHANNEL SYNC"=1852352, "READOUT DIRECTION"=4211904, "PRE HSYNC COUNT"=1852704] ("Parameter")
                w688 = u32 1049104 ("Property ID")
                n41 = call <userlib>:"tm_stopcapture.vi"("error in (no error)"=w690, "Handle in"=w693) -> ("error out"=w691:errorcluster, "Handle out"=w692:u32)  [unwired: 8 in]
                n42 = call <userlib>:"tm_unpreparecapture.vi"("error in (no error)"=w691, "Handle in"=w692) -> ("error out"=w679:errorcluster, "Handle out"=w687:u32)  [unwired: 8 in]
                n43 = local read "Trigger Mode"() -> (w689:sgl)
                n44 = call <userlib>:"tm_setpropertyvalue.vi"("error in (no error)"=w679, "Value in"=w689, "Property ID"=w688, "Handle in"=w687) -> ("error out"=w680:errorcluster)  [unwired: 6 in, 1 out]
                n45 = local read "Readout Direction"() -> (w684:sgl)
                n46 = call <userlib>:"tm_getpropertyvalue.vi"("error in (no error)"=w680, "Property ID"=w688, "Handle in"=w687) -> ("error out"=w681:errorcluster, "Value in"=w686:sgl, "Handle out"=w685:u32)  [unwired: 6 in]
                n47 = call <userlib>:"tm_setparameter_a.vi"("error in (no error)"=w681, "Value in"=w684, "Parameter"=w677, "Handle in"=w685) -> ("error out"=w682:errorcluster, "Handle out"=w683:u32)  [unwired: 6 in]
                n48 = local write "Trigger Mode"(w686) -> ()
                n49 = local read "Camera Readout Mode"() -> (w673:u16)
                n50 = call <userlib>:"tm_getparameter_a.vi"("error in (no error)"=w682, "Parameter"=w677, "Handle in"=w683) -> ("error out"=w675:errorcluster, "Value out"=w678:dbl, "Handle out"=w676:u32)  [unwired: 6 in]
                n51 = local write "Readout Direction"(w678) -> ()
                n52 = call <userlib>:"tm_setpropertyvalue.vi"("error in (no error)"=w675, "Value in"=w673, "Property ID"=u32 4194832, "Handle in"=w676) -> ("error out"=w671:errorcluster, "Handle out"=w672:u32)  [unwired: 6 in]
                n53 = case shown="12" w673 {
                  tunnel: [w697 w701] -> w670
                  tunnel: w672 -> [w696 w702]
                  tunnel: w671 -> [w695 w701]
                  tunnel: [w694 w700] -> w668
                  frame 1, Default {
                    n54 = local read "Exposure"() -> (w698:dbl)
                    n55 = call <userlib>:"tm_setpropertyvalue.vi"("error in (no error)"=w695, "Value in"=w698, "Property ID"=u32 2031888, "Handle in"=w696) -> ("error out"=w697:errorcluster, "Handle out"=w694:u32)  [unwired: 6 in]
                  }
                  frame 12 {
                    n56 = local read "Exposure"() -> (w710:dbl)
                    n57 = local read "SVW"() -> (w708:i32)
                    n58 = formula code="slitExpos=frameInter*LW/(LinesToReadout\n+10+LW);\nlineInter = slitExpos / LW;"("frameInter"=w710, "LW"="Slit Width / Lines 2", "LinesToReadout"=w708) -> ("slitExpos"=w703:dbl, "lineInter"=w706:dbl)
                    n59 = call <userlib>:"tm_setpropertyvalue.vi"("Value in"=w706, "Property ID"=u32 4208720, "Handle in"=w702) -> ("Handle out"=w705:u32)  [unwired: 7 in, 1 out]
                    n60 = call <userlib>:"tm_setpropertyvalue.vi"("Value in"=w703, "Property ID"=u32 2031888, "Handle in"=w705) -> ("Handle out"=w700:u32)  [unwired: 7 in, 1 out]
                  }
                }
                n61 = local read "Scan Mode"() -> (w667:dbl)
                n62 = call <userlib>:"tm_setparameter_a.vi"("error in (no error)"=w670, "Value in"=w667, "Parameter"=w664, "Handle in"=w668) -> ("error out"=w669:errorcluster, "Handle out"=w665:u32)  [unwired: 6 in]
                n63 = call <userlib>:"tm_getparameter_a.vi"("error in (no error)"=w669, "Parameter"=w664, "Handle in"=w665) -> ("error out"=w663:errorcluster, "Value out"=w666:dbl, "Handle out"=w662:u32)  [unwired: 6 in]
                n64 = local write "Scan Mode"(w666) -> ()
                n65 = local read "Binning"() -> (w661:u16)
                n66 = call <userlib>:"tm_setparameter_a.vi"("error in (no error)"=w663, "Value in"=w661, "Parameter"=w637, "Handle in"=w662) -> ("error out"=w640:errorcluster, "Handle out"=w639:u32)  [unwired: 6 in]
                n67 = call <userlib>:"tm_getparameter_a.vi"("error in (no error)"=w640, "Parameter"=w637, "Handle in"=w639) -> ("error out"=w636:errorcluster, "Value out"=w638:dbl, "Handle out"=w624:u32)  [unwired: 6 in]
                n68 = local write "Binning"(w638) -> ()
                n69 = local read "V Width"() -> (w626:i32)
                n70 = local read "V Offset"() -> (w628:i32)
                n71 = local read "H Width"() -> (w627:i32)
                n72 = local read "H Offset"() -> (w629:i32)
                n73 = Bundle("H Offset"=w629, "V Offset"=w628, "H Width"=w627, "V Width"=w626) -> (w625:T8)  [unwired: 1 in]
                n74 = call <userlib>:"tm_setarea.vi"("Sub Region"=w625, "Handle in"=w624) -> ("Handle out"=w623:u32)  [unwired: 8 in, 1 out]
                n75 = call <userlib>:"tm_getarea_a.vi"("error in (no error)"=w636, "Handle in"=w623) -> ("error out"=w635:errorcluster, "V Offset"=w643:T6, "H Offset"=w644:T6, "Handle out"=w622:u32, "H Width"=w642:T6, "V Width"=w641:T6)  [unwired: 4 in]
                n76 = Unbundle By Name(w644) -> ("Value"=w648:i32, "Minimum"=w645:i32, "Maximum"=w646:i32, "Increment"=w647:i32)
                n77 = Unbundle By Name(w643) -> ("Value"=w658:i32, "Minimum"=w649:i32, "Maximum"=w650:i32, "Increment"=w651:i32)
                n78 = Unbundle By Name(w642) -> ("Value"=w659:i32, "Minimum"=w652:i32, "Maximum"=w653:i32, "Increment"=w654:i32)
                n79 = Unbundle By Name(w641) -> ("Value"=w660:i32, "Minimum"=w655:i32, "Maximum"=w656:i32, "Increment"=w657:i32)
                n80 = property on="H Offset" class="DigNum (strict)"("Value"=w648, "Minimum"=w645, "Maximum"=w646, "Increment"=w647) -> ()  [unwired: 2 in, 2 out]
                n81 = property on="V Offset" class="DigNum (strict)"("Value"=w658, "Minimum"=w649, "Maximum"=w650, "Increment"=w651) -> ()  [unwired: 2 in, 2 out]
                n82 = property on="H Width" class="DigNum (strict)"("Value"=w659, "Minimum"=w652, "Maximum"=w653, "Increment"=w654) -> ()  [unwired: 2 in, 2 out]
                n83 = property on="V Width" class="DigNum (strict)"("Value"=w660, "Minimum"=w655, "Maximum"=w656, "Increment"=w657) -> ()  [unwired: 2 in, 2 out]
                n84 = local write "SHO"(w648) -> ()
                n85 = local write "SVO"(w658) -> ()
                n86 = local write "SHW"(w659) -> ()
                n87 = local write "SVW"(w660) -> ()
                n88 = call <userlib>:"tm_preparecapture.vi"("error in (no error)"=w635, "Capture mode"=w634, "Handle in"=w622) -> ("error out"=w633:errorcluster, "Buffer Info"=w631:T7, "Handle out"=w632:u32)  [unwired: 5 in, 1 out]
                n89 = call <userlib>:"tm_startcapture_b.vi"("error in (no error)"=w633, "Handle in"=w632) -> ("error out"=w630:errorcluster, "Handle out"=w621:u32)  [unwired: 8 in]
              }
              frame "Update" {
                w721 = u32 1066144 items=["SENSOR MODE"=4212128, "CCD MODE"=4212384, "READOUT MODE"=4211872, "ACTIVE VIEW INDEX"=4343136, "BITS PER CHANNEL"=4342976, "IMAGE PIXEL TYPE"=4343296, "BINNING"=4215968, "EXPOSURE TIME"=2049184, "CONTRAST GAIN"=3163312, "CONTRAST OFFSET"=3163328, "LIGHT MODE"=2114720, "SENSITIVITY"=2114992, "PHOTON IMAGING MODE"=2115200, "HIGH DYNAMIC RANGE MODE"=3163360, "WHITE BALANCE"=3163568, "TEMPERATURE"=2115232, "TEMPERATURE TARGET"=2115264, "SENSOR COOLER FAN"=2115296, "LINEBUNDLE HEIGHT"=4212192, "MECHANICAL SHUTTER"=2115488, "BACK FOCUS POSITION"=8422304, "TRIGGER CONNECTOR"=1066432, "TRIGGER SOURCE"=1066144, "OUTPUT TRIGGER SOURCE"=1852576, "TRIGGER GLOBAL EXPOSURE"=2049680, "FIRST TRIGGER BEHAVIOR"=2049696, "CHANNEL SYNC"=1852352, "READOUT DIRECTION"=4211904, "PRE HSYNC COUNT"=1852704] ("Parameter")
                w726 = u32 4191424 items=["SENSOR MODE"=4212128, "CCD MODE"=4212384, "READOUT MODE"=4211872, "ACTIVE VIEW INDEX"=4343136, "BITS PER CHANNEL"=4342976, "IMAGE PIXEL TYPE"=4343296, "BINNING"=4215968, "EXPOSURE TIME"=2049184, "CONTRAST GAIN"=3163312, "CONTRAST OFFSET"=3163328, "LIGHT MODE"=2114720, "SENSITIVITY"=2114992, "PHOTON IMAGING MODE"=2115200, "HIGH DYNAMIC RANGE MODE"=3163360, "WHITE BALANCE"=3163568, "TEMPERATURE"=2115232, "TEMPERATURE TARGET"=2115264, "SENSOR COOLER FAN"=2115296, "LINEBUNDLE HEIGHT"=4212192, "MECHANICAL SHUTTER"=2115488, "BACK FOCUS POSITION"=8422304, "TRIGGER CONNECTOR"=1066432, "TRIGGER SOURCE"=1066144, "OUTPUT TRIGGER SOURCE"=1852576, "TRIGGER GLOBAL EXPOSURE"=2049680, "FIRST TRIGGER BEHAVIOR"=2049696, "CHANNEL SYNC"=1852352, "READOUT DIRECTION"=4211904, "PRE HSYNC COUNT"=1852704, "INTERNAL LINE SPEED"=4191408, "INTERNAL LINE INVERVAL"=4191424] ("Parameter")
                w727 = u32 2049184 items=["SENSOR MODE"=4212128, "CCD MODE"=4212384, "READOUT MODE"=4211872, "ACTIVE VIEW INDEX"=4343136, "BITS PER CHANNEL"=4342976, "IMAGE PIXEL TYPE"=4343296, "BINNING"=4215968, "EXPOSURE TIME"=2049184, "CONTRAST GAIN"=3163312, "CONTRAST OFFSET"=3163328, "LIGHT MODE"=2114720, "SENSITIVITY"=2114992, "PHOTON IMAGING MODE"=2115200, "HIGH DYNAMIC RANGE MODE"=3163360, "WHITE BALANCE"=3163568, "TEMPERATURE"=2115232, "TEMPERATURE TARGET"=2115264, "SENSOR COOLER FAN"=2115296, "LINEBUNDLE HEIGHT"=4212192, "MECHANICAL SHUTTER"=2115488, "BACK FOCUS POSITION"=8422304, "TRIGGER CONNECTOR"=1066432, "TRIGGER SOURCE"=1066144, "OUTPUT TRIGGER SOURCE"=1852576, "TRIGGER GLOBAL EXPOSURE"=2049680, "FIRST TRIGGER BEHAVIOR"=2049696, "CHANNEL SYNC"=1852352, "READOUT DIRECTION"=4211904, "PRE HSYNC COUNT"=1852704] ("Parameter")
                n90 = local read "EXP"() -> (w732:dbl)
                n91 = call <userlib>:"tm_setparameter_a.vi"("error in (no error)"=w730, "Value in"=w732, "Parameter"=w727, "Handle in"=w731) -> ("error out"=w734:errorcluster, "Handle out"=w728:u32)  [unwired: 6 in]
                n92 = call <userlib>:"tm_getparameter_a.vi"("error in (no error)"=w734, "Parameter"=w727, "Handle in"=w728) -> ("error out"=w711:errorcluster, "Value out"=w733:dbl, "Handle out"=w729:u32)  [unwired: 6 in]
                n93 = local read "Internal Line Interval"() -> (w719:dbl)
                n94 = local write "EXP"(w733) -> ()
                n95 = call <userlib>:"tm_setparameter_a.vi"("error in (no error)"=w711, "Value in"=w719, "Parameter"=w726, "Handle in"=w729) -> ("error out"=w712:errorcluster, "Handle out"=w725:u32)  [unwired: 6 in]
                n96 = call <userlib>:"tm_getparameter_a.vi"("error in (no error)"=w712, "Parameter"=w726, "Handle in"=w725) -> ("error out"=w713:errorcluster, "Value out"=w724:dbl, "Handle out"=w723:u32)  [unwired: 6 in]
                n97 = local write "Internal Line Interval"(w724) -> ()
                n98 = local read "Trigger Source"() -> (w718:sgl)
                n99 = call <userlib>:"tm_setparameter_a.vi"("error in (no error)"=w713, "Value in"=w718, "Parameter"=w721, "Handle in"=w723) -> ("error out"=w714:errorcluster, "Handle out"=w722:u32)  [unwired: 6 in]
                n100 = call <userlib>:"tm_getparameter_a.vi"("error in (no error)"=w714, "Parameter"=w721, "Handle in"=w722) -> ("error out"=w715:errorcluster, "Value out"=w720:dbl, "Handle out"=w717:u32)  [unwired: 6 in]
                n101 = local write "Trigger Source"(w720) -> ()
              }
              frame "Idle", Default {
                n102 = call <userlib>:"tm_waitnextframe.vi"("error in (no error)"=w736, "Timeout"=100, "Handle in"=w748) -> ("error out"=w735:errorcluster, "Handle out"=w747:u32)  [unwired: 5 in, 2 out]
                n103 = call <userlib>:"tm_getframe_a.vi"("error in (no error)"=w735, "Buffer Info"=w740, "Handle in"=w747) -> ("error out"=w738:errorcluster, "Data 16"=w742:u16[][], "Handle out"=w739:u32)  [unwired: 4 in, 2 out]
                n104 = Bundle By Name(cluster=w745, "State"=Stack_Track."Idle", "Stack Number"=0, "Image"=w742) -> (w741:cluster{})
                n105 = Enqueue Element(queue=w746, element=w741) -> ()  [unwired: 2 in, 3 out]
              }
            }
            n106 = local read "stop"() -> (w599:bool)
          }
          n107 = while {
            tunnel: w587 -> [w596]
            stop <- "stop" stop-if-true
            n108 = event shown="[0] Timeout" {
              selector: _ -> [_]
              dyn-events: _ -> [_]
              timeout: _ -> [_]
              tunnel: w596 -> [w598]
              event Timeout {
                n109 = event-data() -> ()  [unwired: 1 in, 3 out]
                n110 = Enqueue Element(queue=w598, element=CameraControlTypeDef."Idle") -> ()  [unwired: 2 in, 3 out]
              }
            }
          }
        }
        frame Enabled {
        }
      }
      n111 = while {
        tunnel: w81 -> [w101]
        tunnel: [w99] -> _
        tunnel: [w98] -> w9
        shift-right: [w108] -> _
        shift-left: w80 -> [w106]
        shift-right: [w109] -> _
        shift-left: 0.0 -> [w107]
        shift-right: [w100] -> w10
        shift-left: w80 -> [w104]
        tunnel: w14 -> [w102]
        tunnel: w80 -> [w105]
        shift-right: [w97] -> _
        shift-left: w13 -> [w103]
        shift-right: [w95] -> _
        shift-left: 0 -> [w96]
        tunnel: w15 -> [w94]
        shift-right: [w92] -> _
        shift-left: _ -> [w91]
        tunnel: w12 -> [w90]
        stop <- w110 stop-if-true
        n112 = event shown="[4] \"Trigger Mode\": Value Change" {
          selector: _ -> [_ _ _ _ _ _ _ _ _ _ _ _]
          dyn-events: _ -> [_ _ _ _ _ _ _ _ _ _ _ _]
          timeout: 0 -> [_ _ _ _ _ _ _ _ _ _ _ _]
          tunnel: [w121 w190 w204 w217 w236 w256 w278 w306 w403 w497 w533 w578] -> w109
          tunnel: [w120 w191 w205 w218 w237 w257 w279 w307 w404 w498 w534 w579] -> w108
          tunnel: w107 -> [w132 w190 w204 w217 w236 w256 w278 w306 w403 w497 w533 w578]
          tunnel: w106 -> [w123 w191 w205 w218 w237 w257 w279 w307 w404 w498 w534 w579]
          tunnel: w105 -> [w128 _ _ _ _ _ _ _ _ _ _ _]
          tunnel: w104 -> [w133 w192 w206 w219 w238 w258 w280 w302 w399 w499 w541 w586]
          tunnel: w103 -> [w127 w189 w203 w216 _ w255 _ w303 w400 _ _ _]
          tunnel: w102 -> [w135 w185 w198 w212 w231 w249 w271 w310 w407 w494 w510 w548]
          tunnel: w101 -> [w134 w187 w194 w213 w230 w252 w270 w311 w408 w493 w509 w547]
          tunnel: [w131 w192 w206 w219 w238 w258 w280 w302 w399 w499 w541 w586] -> w100
          tunnel: [w130 w182 w201 w209 w222 w242 w261 w308 w405 w488 w536 w581] -> w99
          tunnel: [w129 w181 w200 w208 w221 w241 w259 w309 w406 w489 w537 w582] -> w98
          tunnel: [w126 w189 w203 w216 w225 w255 w266 w304 w401 w487 w535 w580] -> w97
          tunnel: w96 -> [w118 w188 w202 w215 w235 w254 w277 w305 w402 w486 w506 w542]
          tunnel: [w117 w188 w202 w215 w235 w254 w277 w305 w402 w486 w506 w542] -> w95
          tunnel: w94 -> [w112 _ _ _ _ _ _ w301 w398 _ _ _]
          tunnel: [_ _ _ _ _ _ _ w300 w397 _ _ _] -> w93
          tunnel: w90 -> [w115 _ _ _ _ _ _ w298 _ _ _ _]
          tunnel: [w114 _ _ _ _ _ _ _ _ _ _ _] -> w92
          tunnel: w91 -> [w113 _ _ _ _ _ _ w299 _ _ _ _]
          event Timeout {
            n113 = event-data() -> ()  [unwired: 1 in, 2 out]
            n114 = call <userlib>:"tm_waitnextframe.vi"("error in (no error)"=w134, "Handle in"=w135) -> ("error out"=w138:errorcluster, "Frame Count"=w119:i32, "Frame Index"=w137:i32, "Handle out"=w139:u32)  [unwired: 6 in]
            "Total Frames" <- w119
            n115 = Tick Count (ms)() -> (millisecond timer value=w125:u32)
            n116 = Increment(x=w132) -> (x+1=w122:dbl)
            n117 = Subtract(x=w125, y=w128) -> (x-y=→"Elapsed Time":u32)
            n118 = Add(x=w123, y=u32 1000) -> (x+y=w143:u32)
            n119 = Less Or Equal?(x=w143, y=w125) -> (x <= y?=w124:bool)
            n120 = Add(x=w133, y=u32 50) -> (x+y=w141:u32)
            n121 = Less Or Equal?(x=w141, y=w125) -> (x <= y?=w116:bool)
            n122 = case shown="True" w124 {
              tunnel: w123 -> [w146 w155]
              tunnel: [w146 w152] -> w120
              tunnel: w122 -> [w145 w158]
              tunnel: w125 -> [_ w152]
              tunnel: [w145 0.0] -> w121
              tunnel: w119 -> [_ w147]
              tunnel: w118 -> [w144 w150]
              tunnel: [w144 w147] -> w117
              frame False {
              }
              frame True {
                n123 = Subtract(x=w152, y=w155) -> (x-y=w154:u32)
                n124 = Subtract(x=w147, y=w150) -> (x-y=w148:i32)
                n125 = To Double Precision Float(number=w154) -> (double precision float=w160:dbl)
                n126 = Divide(x=w160, y=1000.0) -> (x/y=w151:dbl)
                n127 = To Double Precision Float(number=w148) -> (double precision float=w149:dbl)
                n128 = Divide(x=w149, y=w151) -> (x/y=→"Camera FPS":dbl)
                n129 = Divide(x=w158, y=w151) -> (x/y=→"Software FPS":dbl)
              }
            }
            n130 = case shown="True" w116 {
              tunnel: w133 -> [w165 _]
              tunnel: w125 -> [_ w178]
              tunnel: [w165 w178] -> w131
              tunnel: w139 -> [w164 w177]
              tunnel: w127 -> [w162 w172]
              tunnel: w138 -> [w163 w176]
              tunnel: [w164 w175] -> w130
              tunnel: [w163 w174] -> w129
              tunnel: w137 -> [_ w173]
              tunnel: [w162 w172] -> w126
              tunnel: w112 -> [_ w171]
              tunnel: w115 -> [_ w167]
              tunnel: [w161 w166] -> w114
              tunnel: w113 -> [w161 _]
              frame False {
              }
              frame True {
                n131 = call <userlib>:"tm_getframe_a.vi"("error in (no error)"=w176, "Frame Index"=w173, "Buffer Info"=w172, "Handle in"=w177) -> ("error out"=w174:errorcluster, "Data 16"=w166:u16[][], "Handle out"=w175:u32)  [unwired: 3 in, 2 out]
                "Image 2" <- w166
                n132 = Bundle By Name(cluster=w167, "State"=Stack_Track."Idle", "Stack Number"=0, "Image"=w166) -> (w168:T2)
                n133 = Enqueue Element(queue=w171, element=w168) -> ()  [unwired: 2 in, 3 out]
              }
            }
          }
          event "Exposure": Value Change {
            w180 = u32 2049184 items=["SENSOR MODE"=4212128, "CCD MODE"=4212384, "READOUT MODE"=4211872, "ACTIVE VIEW INDEX"=4343136, "BITS PER CHANNEL"=4342976, "IMAGE PIXEL TYPE"=4343296, "BINNING"=4215968, "EXPOSURE TIME"=2049184, "CONTRAST GAIN"=3163312, "CONTRAST OFFSET"=3163328, "LIGHT MODE"=2114720, "SENSITIVITY"=2114992, "PHOTON IMAGING MODE"=2115200, "HIGH DYNAMIC RANGE MODE"=3163360, "WHITE BALANCE"=3163568, "TEMPERATURE"=2115232, "TEMPERATURE TARGET"=2115264, "SENSOR COOLER FAN"=2115296, "LINEBUNDLE HEIGHT"=4212192, "MECHANICAL SHUTTER"=2115488, "BACK FOCUS POSITION"=8422304, "TRIGGER CONNECTOR"=1066432, "TRIGGER SOURCE"=1066144, "OUTPUT TRIGGER SOURCE"=1852576, "TRIGGER GLOBAL EXPOSURE"=2049680, "FIRST TRIGGER BEHAVIOR"=2049696, "CHANNEL SYNC"=1852352, "READOUT DIRECTION"=4211904, "PRE HSYNC COUNT"=1852704] ("Parameter")
            n134 = event-data() -> ("NewVal"=w186:dbl)  [unwired: 1 in, 2 out]
            n135 = call <userlib>:"tm_setparameter_a.vi"("error in (no error)"=w187, "Value in"=w186, "Parameter"=w180, "Handle in"=w185) -> ("error out"=w184:errorcluster, "Handle out"=w183:u32)  [unwired: 6 in]
            n136 = call <userlib>:"tm_getparameter_a.vi"("error in (no error)"=w184, "Parameter"=w180, "Handle in"=w183) -> ("error out"=w181:errorcluster, "Value out"=w179:dbl, "Handle out"=w182:u32)  [unwired: 6 in]
            n137 = local write "EXP"(w179) -> ()
          }
          event "Internal Line Interval": Value Change {
            w193 = u32 4191424 items=["SENSOR MODE"=4212128, "CCD MODE"=4212384, "READOUT MODE"=4211872, "ACTIVE VIEW INDEX"=4343136, "BITS PER CHANNEL"=4342976, "IMAGE PIXEL TYPE"=4343296, "BINNING"=4215968, "EXPOSURE TIME"=2049184, "CONTRAST GAIN"=3163312, "CONTRAST OFFSET"=3163328, "LIGHT MODE"=2114720, "SENSITIVITY"=2114992, "PHOTON IMAGING MODE"=2115200, "HIGH DYNAMIC RANGE MODE"=3163360, "WHITE BALANCE"=3163568, "TEMPERATURE"=2115232, "TEMPERATURE TARGET"=2115264, "SENSOR COOLER FAN"=2115296, "LINEBUNDLE HEIGHT"=4212192, "MECHANICAL SHUTTER"=2115488, "BACK FOCUS POSITION"=8422304, "TRIGGER CONNECTOR"=1066432, "TRIGGER SOURCE"=1066144, "OUTPUT TRIGGER SOURCE"=1852576, "TRIGGER GLOBAL EXPOSURE"=2049680, "FIRST TRIGGER BEHAVIOR"=2049696, "CHANNEL SYNC"=1852352, "READOUT DIRECTION"=4211904, "PRE HSYNC COUNT"=1852704, "INTERNAL LINE SPEED"=4191408, "INTERNAL LINE INVERVAL"=4191424] ("Parameter")
            n138 = event-data() -> ("NewVal"=w197:dbl)  [unwired: 1 in, 2 out]
            n139 = call <userlib>:"tm_setparameter_a.vi"("error in (no error)"=w194, "Value in"=w197, "Parameter"=w193, "Handle in"=w198) -> ("error out"=w195:errorcluster, "Handle out"=w196:u32)  [unwired: 6 in]
            n140 = call <userlib>:"tm_getparameter_a.vi"("error in (no error)"=w195, "Parameter"=w193, "Handle in"=w196) -> ("error out"=w200:errorcluster, "Value out"=w199:dbl, "Handle out"=w201:u32)  [unwired: 6 in]
            n141 = local write "Internal Line Interval"(w199) -> ()
          }
          event "Trigger Source": Value Change {
            w214 = u32 1066144 items=["SENSOR MODE"=4212128, "CCD MODE"=4212384, "READOUT MODE"=4211872, "ACTIVE VIEW INDEX"=4343136, "BITS PER CHANNEL"=4342976, "IMAGE PIXEL TYPE"=4343296, "BINNING"=4215968, "EXPOSURE TIME"=2049184, "CONTRAST GAIN"=3163312, "CONTRAST OFFSET"=3163328, "LIGHT MODE"=2114720, "SENSITIVITY"=2114992, "PHOTON IMAGING MODE"=2115200, "HIGH DYNAMIC RANGE MODE"=3163360, "WHITE BALANCE"=3163568, "TEMPERATURE"=2115232, "TEMPERATURE TARGET"=2115264, "SENSOR COOLER FAN"=2115296, "LINEBUNDLE HEIGHT"=4212192, "MECHANICAL SHUTTER"=2115488, "BACK FOCUS POSITION"=8422304, "TRIGGER CONNECTOR"=1066432, "TRIGGER SOURCE"=1066144, "OUTPUT TRIGGER SOURCE"=1852576, "TRIGGER GLOBAL EXPOSURE"=2049680, "FIRST TRIGGER BEHAVIOR"=2049696, "CHANNEL SYNC"=1852352, "READOUT DIRECTION"=4211904, "PRE HSYNC COUNT"=1852704] ("Parameter")
            n142 = event-data() -> ("NewVal"=w207:sgl)  [unwired: 1 in, 3 out]
            n143 = call <userlib>:"tm_setparameter_a.vi"("error in (no error)"=w213, "Value in"=w207, "Parameter"=w214, "Handle in"=w212) -> ("error out"=w211:errorcluster, "Handle out"=w210:u32)  [unwired: 6 in]
            n144 = call <userlib>:"tm_getparameter_a.vi"("error in (no error)"=w211, "Parameter"=w214, "Handle in"=w210) -> ("error out"=w208:errorcluster, "Handle out"=w209:u32)  [unwired: 6 in, 1 out]
          }
          event "Trigger Mode": Value Change {
            w226 = 1 items=["Snap", "Sequence"] ("Capture mode")
            n145 = event-data() -> ("NewVal"=w220:sgl)  [unwired: 1 in, 4 out]
            n146 = call <userlib>:"tm_stopcapture.vi"("error in (no error)"=w230, "Handle in"=w231) -> ("error out"=w233:errorcluster, "Handle out"=w232:u32)  [unwired: 8 in]
            n147 = call <userlib>:"tm_unpreparecapture.vi"("error in (no error)"=w233, "Handle in"=w232) -> ("error out"=w229:errorcluster, "Handle out"=w228:u32)  [unwired: 8 in]
            n148 = call <userlib>:"tm_setpropertyvalue.vi"("error in (no error)"=w229, "Value in"=w220, "Property ID"=u32 1049104, "Handle in"=w228) -> ("error out"=w224:errorcluster, "Handle out"=w227:u32)  [unwired: 6 in]
            n149 = call <userlib>:"tm_preparecapture.vi"("Capture mode"=w226, "Handle in"=w227) -> ("Buffer Info"=w225:T7, "Handle out"=w223:u32)  [unwired: 6 in, 2 out]
            n150 = call <userlib>:"tm_startcapture_b.vi"("error in (no error)"=w224, "Handle in"=w223) -> ("error out"=w221:errorcluster, "Handle out"=w222:u32)  [unwired: 8 in]
          }
          event "Readout Direction": Value Change {
            w247 = 1 items=["Snap", "Sequence"] ("Capture mode")
            w240 = u32 4211904 items=["SENSOR MODE"=4212128, "CCD MODE"=4212384, "READOUT MODE"=4211872, "ACTIVE VIEW INDEX"=4343136, "BITS PER CHANNEL"=4342976, "IMAGE PIXEL TYPE"=4343296, "BINNING"=4215968, "EXPOSURE TIME"=2049184, "CONTRAST GAIN"=3163312, "CONTRAST OFFSET"=3163328, "LIGHT MODE"=2114720, "SENSITIVITY"=2114992, "PHOTON IMAGING MODE"=2115200, "HIGH DYNAMIC RANGE MODE"=3163360, "WHITE BALANCE"=3163568, "TEMPERATURE"=2115232, "TEMPERATURE TARGET"=2115264, "SENSOR COOLER FAN"=2115296, "LINEBUNDLE HEIGHT"=4212192, "MECHANICAL SHUTTER"=2115488, "BACK FOCUS POSITION"=8422304, "TRIGGER CONNECTOR"=1066432, "TRIGGER SOURCE"=1066144, "OUTPUT TRIGGER SOURCE"=1852576, "TRIGGER GLOBAL EXPOSURE"=2049680, "FIRST TRIGGER BEHAVIOR"=2049696, "CHANNEL SYNC"=1852352, "READOUT DIRECTION"=4211904, "PRE HSYNC COUNT"=1852704] ("Parameter")
            n151 = event-data() -> ("NewVal"=w239:sgl)  [unwired: 1 in, 3 out]
            n152 = call <userlib>:"tm_stopcapture.vi"("error in (no error)"=w252, "Handle in"=w249) -> ("error out"=w253:errorcluster, "Handle out"=w248:u32)  [unwired: 8 in]
            n153 = call <userlib>:"tm_unpreparecapture.vi"("error in (no error)"=w253, "Handle in"=w248) -> ("error out"=w251:errorcluster, "Handle out"=w250:u32)  [unwired: 8 in]
            n154 = call <userlib>:"tm_setparameter_a.vi"("error in (no error)"=w251, "Value in"=w239, "Parameter"=w240, "Handle in"=w250) -> ("error out"=w244:errorcluster, "Handle out"=w243:u32)  [unwired: 6 in]
            n155 = call <userlib>:"tm_preparecapture.vi"("error in (no error)"=w244, "Capture mode"=w247, "Handle in"=w243) -> ("error out"=w245:errorcluster, "Handle out"=w246:u32)  [unwired: 5 in, 2 out]
            n156 = call <userlib>:"tm_startcapture_b.vi"("error in (no error)"=w245, "Handle in"=w246) -> ("error out"=w241:errorcluster, "Handle out"=w242:u32)  [unwired: 8 in]
          }
          event "Camera Readout Mode", "Slit Width / Lines": Value Change {
            w264 = 1 items=["Snap", "Sequence"] ("Capture mode")
            n157 = event-data() -> ()  [unwired: 1 in, 4 out]
            n158 = call <userlib>:"tm_stopcapture.vi"("error in (no error)"=w270, "Handle in"=w271) -> ("error out"=w272:errorcluster, "Handle out"=w268:u32)  [unwired: 8 in]
            n159 = call <userlib>:"tm_unpreparecapture.vi"("error in (no error)"=w272, "Handle in"=w268) -> ("error out"=w263:errorcluster, "Handle out"=w269:u32)  [unwired: 8 in]
            n160 = call <userlib>:"tm_setpropertyvalue.vi"("error in (no error)"=w263, "Value in"="Camera Readout Mode", "Property ID"=u32 4194832, "Handle in"=w269) -> ("error out"=w273:errorcluster, "Handle out"=w274:u32)  [unwired: 6 in]
            n161 = case shown="12" "Camera Readout Mode" {
              tunnel: w274 -> [w285 w292]
              tunnel: [w284 w287] -> w267
              tunnel: w273 -> [w282 w297]
              tunnel: [w281 w297] -> w265
              frame 1, Default {
                n162 = local read "Exposure"() -> (w283:dbl)
                n163 = call <userlib>:"tm_setpropertyvalue.vi"("error in (no error)"=w282, "Value in"=w283, "Property ID"=u32 2031888, "Handle in"=w285) -> ("error out"=w281:errorcluster, "Handle out"=w284:u32)  [unwired: 6 in]
              }
              frame 12 {
                n164 = local read "Exposure"() -> (w296:dbl)
                n165 = local read "SVW"() -> (w294:i32)
                n166 = formula code="slitExpos=frameInter*LW/(LinesToReadout\n+10+LW);\nlineInter = slitExpos / LW;"("frameInter"=w296, "LW"="Slit Width / Lines", "LinesToReadout"=w294) -> ("slitExpos"=w288:dbl, "lineInter"=w291:dbl)
                n167 = call <userlib>:"tm_setpropertyvalue.vi"("Value in"=w291, "Property ID"=u32 4208720, "Handle in"=w292) -> ("Handle out"=w290:u32)  [unwired: 7 in, 1 out]
                n168 = call <userlib>:"tm_setpropertyvalue.vi"("Value in"=w288, "Property ID"=u32 2031888, "Handle in"=w290) -> ("Handle out"=w287:u32)  [unwired: 7 in, 1 out]
              }
            }
            n169 = call <userlib>:"tm_preparecapture.vi"("error in (no error)"=w265, "Capture mode"=w264, "Handle in"=w267) -> ("error out"=w260:errorcluster, "Buffer Info"=w266:T7, "Handle out"=w262:u32)  [unwired: 5 in, 1 out]
            n170 = call <userlib>:"tm_startcapture_b.vi"("error in (no error)"=w260, "Handle in"=w262) -> ("error out"=w259:errorcluster, "Handle out"=w261:u32)  [unwired: 8 in]
          }
          event "Ram Record": Value Change {
            n171 = event-data() -> ()  [unwired: 1 in, 5 out]
            n172 = case shown="True" "Ram Record" {
              tunnel: w311 -> [w315 w338]
              tunnel: w310 -> [w314 w335]
              tunnel: [w315 w321] -> w309
              tunnel: [w314 w323] -> w308
              tunnel: [w313 w322] -> w304
              tunnel: w303 -> [w313 _]
              tunnel: w301 -> [_ w326]
              tunnel: [_ w324] -> w300
              tunnel: w299 -> [_ w320]
              tunnel: w298 -> [_ w316]
              frame False {
              }
              frame True {
                w332 = 0 items=["Snap", "Sequence"] ("Capture mode")
                # "Max 2500"
                n173 = Flush Queue(queue=w326) -> (queue out=w325:refnum<queue>)  [unwired: 1 in, 2 out]
                n174 = call <userlib>:"tm_stopcapture.vi"("error in (no error)"=w338, "Handle in"=w335) -> ("error out"=w337:errorcluster, "Handle out"=w336:u32)  [unwired: 8 in]
                n175 = call <userlib>:"tm_unpreparecapture.vi"("error in (no error)"=w337, "Handle in"=w336) -> ("error out"=w333:errorcluster, "Handle out"=w334:u32)  [unwired: 8 in]
                n176 = call <userlib>:"tm_preparecapture.vi"("error in (no error)"=w333, "Frames"="Frames", "Capture mode"=w332, "Handle in"=w334) -> ("error out"=w331:errorcluster, "Buffer Info"=w329:T7, "Handle out"=w330:u32)  [unwired: 4 in, 1 out]
                n177 = Bundle By Name(cluster=w316, "State"=Stack_Track."Start Sequence", "Stack Number"=0, "Image"=w320) -> (w317:T2)
                n178 = Enqueue Element(queue=w325, element=w317) -> (queue out=w327:refnum<queue>)  [unwired: 2 in, 2 out]
                n179 = case shown="No Error" w331 {
                  selector: w331 -> [w363 w384]
                  tunnel: w330 -> [w362 w385]
                  tunnel: "Frames" -> [w358 _]
                  tunnel: [w343 w381] -> w323
                  tunnel: w329 -> [w359 _]
                  tunnel: [w342 w383] -> w321
                  tunnel: w327 -> [w357 w379]
                  tunnel: w316 -> [w356 _]
                  tunnel: [w341 w379] -> _
                  tunnel: [FALSE ("value") w393] -> w324
                  tunnel: [w340 w382] -> w322
                  frame No Error {
                    w348 = 1 items=["Snap", "Sequence"] ("Capture mode")
                    # "Frames in RAM"
                    n180 = call <userlib>:"tm_startcapture_b.vi"("error in (no error)"=w363, "Handle in"=w362) -> ("error out"=w360:errorcluster, "Handle out"=w361:u32)  [unwired: 8 in]
                    n181 = for {
                      N: w358 -> [_]
                      tunnel: w361 -> [w378]
                      tunnel: w360 -> [w377]
                      tunnel: w359 -> [w374]
                      tunnel: [w373] -> w354
                      tunnel: [w372] -> w353
                      tunnel: w357 -> [w370]
                      tunnel: Stack_Track."Collecting" ("Enum") -> [w368]
                      tunnel: w356 -> [w366]
                      tunnel: [w365] -> w347
                      i -> [w367]
                      n182 = call <userlib>:"tm_waitnextframe.vi"("error in (no error)"=w377, "Handle in"=w378) -> ("error out"=w375:errorcluster, "Frame Index"=→"Frame Index":i32, "Handle out"=w376:u32)  [unwired: 6 in, 1 out]
                      n183 = call <userlib>:"tm_getframe_a.vi"("error in (no error)"=w375, "Frame Index"=w367, "Buffer Info"=w374, "Handle in"=w376) -> ("error out"=w372:errorcluster, "Data 16"=w364:u16[][], "Handle out"=w373:u32)  [unwired: 3 in, 2 out]
                      n184 = Bundle By Name(cluster=w366, "State"=w368, "Stack Number"=w367, "Image"=w364) -> (w369:T2)
                      n185 = Enqueue Element(queue=w370, element=w369) -> (queue out=w365:refnum<queue>)  [unwired: 2 in, 2 out]
                    }
                    n186 = call <userlib>:"tm_stopcapture.vi"("error in (no error)"=w353, "Handle in"=w354) -> ("error out"=w351:errorcluster, "Handle out"=w352:u32)  [unwired: 8 in]
                    n187 = call <userlib>:"tm_unpreparecapture.vi"("error in (no error)"=w351, "Handle in"=w352) -> ("error out"=w350:errorcluster, "Handle out"=w349:u32)  [unwired: 8 in]
                    n188 = Enqueue Element(queue=w347, element=T2 {"State"=enum."End", "Stack Number"=0, "Image"=[]} ("input cluster")) -> (queue out=w341:refnum<queue>)  [unwired: 2 in, 2 out]
                    n189 = call <userlib>:"tm_preparecapture.vi"("error in (no error)"=w350, "Capture mode"=w348, "Handle in"=w349) -> ("error out"=w345:errorcluster, "Buffer Info"=w340:T7, "Handle out"=w344:u32)  [unwired: 5 in, 1 out]
                    n190 = call <userlib>:"tm_startcapture_b.vi"("error in (no error)"=w345, "Handle in"=w344) -> ("error out"=w342:errorcluster, "Handle out"=w343:u32)  [unwired: 8 in]
                  }
                  frame Error {
                    w388 = 1 items=["Snap", "Sequence"] ("Capture mode")
                    # "Prepare camera failure, likely too many frames in stack"
                    n191 = One Button Dialog(message="Too many frames in stack", button name ("OK")="OK") -> (true=w393:bool)
                    n192 = call <userlib>:"tm_stopcapture.vi"("error in (no error)"=w384, "Handle in"=w385) -> ("error out"=w391:errorcluster, "Handle out"=w392:u32)  [unwired: 8 in]
                    n193 = call <userlib>:"tm_unpreparecapture.vi"("error in (no error)"=w391, "Handle in"=w392) -> ("error out"=w390:errorcluster, "Handle out"=w389:u32)  [unwired: 8 in]
                    n194 = Enqueue Element(queue=w379, element=T2 {"State"=enum."Idle", "Stack Number"=0, "Image"=[]} ("input cluster")) -> ()  [unwired: 2 in, 3 out]
                    n195 = call <userlib>:"tm_preparecapture.vi"("error in (no error)"=w390, "Capture mode"=w388, "Handle in"=w389) -> ("error out"=w387:errorcluster, "Buffer Info"=w382:T7, "Handle out"=w386:u32)  [unwired: 5 in, 1 out]
                    n196 = call <userlib>:"tm_startcapture_b.vi"("error in (no error)"=w387, "Handle in"=w386) -> ("error out"=w383:errorcluster, "Handle out"=w381:u32)  [unwired: 8 in]
                  }
                }
              }
            }
          }
          event "HardDisk Record": Value Change {
            n197 = event-data() -> ()  [unwired: 1 in, 5 out]
            n198 = case shown="True" "HardDisk Record" {
              tunnel: w408 -> [w411 w427]
              tunnel: w407 -> [w410 w424]
              tunnel: [w411 w414] -> w406
              tunnel: [w410 w416] -> w405
              tunnel: [w409 w415] -> w401
              tunnel: w400 -> [w409 _]
              tunnel: w398 -> [_ w412]
              tunnel: [_ w417] -> w397
              frame False {
              }
              frame True {
                w421 = 0 items=["Snap", "Sequence"] ("Capture mode")
                # "Max 50"
                n199 = call <userlib>:"tm_stopcapture.vi"("error in (no error)"=w427, "Handle in"=w424) -> ("error out"=w426:errorcluster, "Handle out"=w425:u32)  [unwired: 8 in]
                n200 = call <userlib>:"tm_unpreparecapture.vi"("error in (no error)"=w426, "Handle in"=w425) -> ("error out"=w422:errorcluster, "Handle out"=w423:u32)  [unwired: 8 in]
                n201 = call <userlib>:"tm_preparecapture.vi"("error in (no error)"=w422, "Frames"="Frames", "Capture mode"=w421, "Handle in"=w423) -> ("error out"=w420:errorcluster, "Buffer Info"=w418:T7, "Handle out"=w419:u32)  [unwired: 4 in, 1 out]
                n202 = case shown="No Error" w420 {
                  selector: w420 -> [w452 w465]
                  tunnel: w419 -> [w438 w466]
                  tunnel: [w441 w462] -> w416
                  tunnel: w418 -> [w449 _]
                  tunnel: [w440 w464] -> w414
                  tunnel: [FALSE ("value") w474] -> w417
                  tunnel: [w439 w463] -> w415
                  tunnel: "Frames" -> [w435 _]
                  tunnel: w412 -> [w429 w460]
                  frame No Error {
                    w444 = 1 items=["Snap", "Sequence"] ("Capture mode")
                    n203 = call <userlib>:"tm_startrecorder.vi"("frames"=w435, "File"="Temp", "Handle in"=w438) -> ("Handle out"=w437:u32)  [unwired: 7 in, 1 out]
                    n204 = call <userlib>:"tm_startcapture_b.vi"("error in (no error)"=w452, "Handle in"=w437) -> ("error out"=w450:errorcluster, "Handle out"=w451:u32)  [unwired: 8 in]
                    n205 = while {
                      tunnel: w451 -> [w458]
                      tunnel: w450 -> [w457]
                      tunnel: w449 -> [_]
                      tunnel: [w459] -> w447
                      tunnel: w435 -> [w454]
                      stop <- w455 stop-if-true
                      n206 = Wait (ms)(milliseconds to wait=u32 50) -> ()  [unwired: 1 out]
                      n207 = call <userlib>:"tm_getrecorderstatus.vi"("error in (no error)"=w457, "Handle"=w458) -> ("error out"=w459:errorcluster, "Count"=w453:i32)  [unwired: 6 in, 2 out]
                      n208 = Equal?(x=w453, y=w454) -> (x = y?=w455:bool)
                    }
                    n209 = call <userlib>:"tm_stopcapture.vi"("error in (no error)"=w447) -> ("error out"=w434:errorcluster, "Handle out"=w433:u32)  [unwired: 9 in]
                    n210 = call <userlib>:"tm_stoprecorder.vi"("error in (no error)"=w434, "Handle in"=w433) -> ("error out"=w431:errorcluster, "Handle out"=w432:u32)  [unwired: 8 in]
                    n211 = Enqueue Element(queue=w429, element=T2 {"State"=enum."Read Disk", "Stack Number"=0, "Image"=[]}, error in (no error)=w431) -> (error out=w430:errorcluster)  [unwired: 1 in, 2 out]
                    n212 = call <userlib>:"tm_unpreparecapture.vi"("error in (no error)"=w430, "Handle in"=w432) -> ("error out"=w446:errorcluster, "Handle out"=w445:u32)  [unwired: 8 in]
                    n213 = call <userlib>:"tm_preparecapture.vi"("error in (no error)"=w446, "Capture mode"=w444, "Handle in"=w445) -> ("error out"=w443:errorcluster, "Buffer Info"=w439:T7, "Handle out"=w442:u32)  [unwired: 5 in, 1 out]
                    n214 = call <userlib>:"tm_startcapture_b.vi"("error in (no error)"=w443, "Handle in"=w442) -> ("error out"=w440:errorcluster, "Handle out"=w441:u32)  [unwired: 8 in]
                  }
                  frame Error {
                    w469 = 1 items=["Snap", "Sequence"] ("Capture mode")
                    # "Prepare camera failure, likely too many frames in stack"
                    n215 = One Button Dialog(message="Too many frames in stack", button name ("OK")="OK") -> (true=w474:bool)
                    n216 = call <userlib>:"tm_stopcapture.vi"("error in (no error)"=w465, "Handle in"=w466) -> ("error out"=w472:errorcluster, "Handle out"=w473:u32)  [unwired: 8 in]
                    n217 = call <userlib>:"tm_unpreparecapture.vi"("error in (no error)"=w472, "Handle in"=w473) -> ("error out"=w471:errorcluster, "Handle out"=w470:u32)  [unwired: 8 in]
                    n218 = Enqueue Element(queue=w460, element=T2 {"State"=enum."STOP", "Stack Number"=0, "Image"=[]} ("input cluster")) -> ()  [unwired: 2 in, 3 out]
                    n219 = call <userlib>:"tm_preparecapture.vi"("error in (no error)"=w471, "Capture mode"=w469, "Handle in"=w470) -> ("error out"=w468:errorcluster, "Buffer Info"=w463:T7, "Handle out"=w467:u32)  [unwired: 5 in, 1 out]
                    n220 = call <userlib>:"tm_startcapture_b.vi"("error in (no error)"=w468, "Handle in"=w467) -> ("error out"=w464:errorcluster, "Handle out"=w462:u32)  [unwired: 8 in]
                  }
                }
              }
            }
          }
          event "Scan Mode": Value Change {
            w477 = u32 4211872 items=["SENSOR MODE"=4212128, "CCD MODE"=4212384, "READOUT MODE"=4211872, "ACTIVE VIEW INDEX"=4343136, "BITS PER CHANNEL"=4342976, "IMAGE PIXEL TYPE"=4343296, "BINNING"=4215968, "EXPOSURE TIME"=2049184, "CONTRAST GAIN"=3163312, "CONTRAST OFFSET"=3163328, "LIGHT MODE"=2114720, "SENSITIVITY"=2114992, "PHOTON IMAGING MODE"=2115200, "HIGH DYNAMIC RANGE MODE"=3163360, "WHITE BALANCE"=3163568, "TEMPERATURE"=2115232, "TEMPERATURE TARGET"=2115264, "SENSOR COOLER FAN"=2115296, "LINEBUNDLE HEIGHT"=4212192, "MECHANICAL SHUTTER"=2115488, "BACK FOCUS POSITION"=8422304, "TRIGGER CONNECTOR"=1066432, "TRIGGER SOURCE"=1066144, "OUTPUT TRIGGER SOURCE"=1852576, "TRIGGER GLOBAL EXPOSURE"=2049680, "FIRST TRIGGER BEHAVIOR"=2049696, "CHANNEL SYNC"=1852352, "READOUT DIRECTION"=4211904, "PRE HSYNC COUNT"=1852704] ("Parameter")
            w492 = 1 items=["Snap", "Sequence"] ("Capture mode")
            n221 = event-data() -> ("NewVal"=w482:dbl)  [unwired: 1 in, 2 out]
            n222 = call <userlib>:"tm_stopcapture.vi"("error in (no error)"=w493, "Handle in"=w494) -> ("error out"=w495:errorcluster, "Handle out"=w496:u32)  [unwired: 8 in]
            n223 = call <userlib>:"tm_unpreparecapture.vi"("error in (no error)"=w495, "Handle in"=w496) -> ("error out"=w480:errorcluster, "Handle out"=w481:u32)  [unwired: 8 in]
            n224 = call <userlib>:"tm_setparameter_a.vi"("error in (no error)"=w480, "Value in"=w482, "Parameter"=w477, "Handle in"=w481) -> ("error out"=w479:errorcluster, "Handle out"=w478:u32)  [unwired: 6 in]
            n225 = call <userlib>:"tm_getparameter_a.vi"("error in (no error)"=w479, "Parameter"=w477, "Handle in"=w478) -> ("error out"=w485:errorcluster, "Value out"=w484:dbl, "Handle out"=w483:u32)  [unwired: 6 in]
            n226 = local write "SMD"(w484) -> ()
            n227 = call <userlib>:"tm_preparecapture.vi"("error in (no error)"=w485, "Capture mode"=w492, "Handle in"=w483) -> ("error out"=w490:errorcluster, "Buffer Info"=w487:T7, "Handle out"=w491:u32)  [unwired: 5 in, 1 out]
            n228 = call <userlib>:"tm_startcapture_b.vi"("error in (no error)"=w490, "Handle in"=w491) -> ("error out"=w489:errorcluster, "Handle out"=w488:u32)  [unwired: 8 in]
          }
          event "Binning": Value Change {
            w501 = u32 4215968 items=["BINNING"=4215968, "BITS PER CHANNEL"=2, "ACTIVE VIEW INDEX"=3, "CCD MODE"=4, "SENSOR MODE"=5, "READOUT MODE"=6, "EXPOSURE TIME"=7, "CONTRAST GAIN"=8, "CONTRAST OFFSET"=9, "LIGHT MODE"=10, "SENSITIVITY"=11, "WHITE BALANCE"=12, "PHOTON IMAGING MODE"=13, "HIGH DYNAMIC RANGE MODE"=14, "TRIGGER SOURCE"=15, "TRIGGER ACTIVE"=16, "TRIGGER MODE"=17, "TRIGGER POLARITY"=18, "TRIGGER GLOBAL EXPOSURE"=19, "FIRST TRIGGER BEHAVIOR"=20, "TRIGGER TIMES"=21, "OUTPUT TRIGGER POLARITY"=22, "OUTPUT TRIGGER DELAY"=23, "OUTPUT TRIGGER PERIOD"=24, "TEMPERATURE"=25, "TEMPERATURE TARGET"=26, "SENSOR COOLER FAN"=27, "MECHANICAL SHUTTER"=28, "BACK FOCUS POSITION"=29, "FRAMEBUNDLE MODE"=30, "FRAMEBUNDLE NUMBER"=31, "LINEBUNDLE HEIGHT"=32, "TRIGGER CONNECTOR"=33, "IMAGE PIXEL TYPE"=34, "OUTPUT TRIGGER KIND"=35, "READOUT DIRECTION"=36, "CHANNEL SYNC"=37] ("Parameter")
            w540 = 1 items=["Snap", "Sequence"] ("Capture mode")
            n229 = event-data() -> ("NewVal"=w502:u16)  [unwired: 1 in, 2 out]
            n230 = call <userlib>:"tm_stopcapture.vi"("error in (no error)"=w509, "Handle in"=w510) -> ("error out"=w507:errorcluster, "Handle out"=w508:u32)  [unwired: 8 in]
            n231 = call <userlib>:"tm_unpreparecapture.vi"("error in (no error)"=w507, "Handle in"=w508) -> ("error out"=w503:errorcluster, "Handle out"=w500:u32)  [unwired: 8 in]
            n232 = call <userlib>:"tm_setparameter_a.vi"("error in (no error)"=w503, "Value in"=w502, "Parameter"=w501, "Handle in"=w500) -> ("error out"=w504:errorcluster, "Handle out"=w505:u32)  [unwired: 6 in]
            n233 = call <userlib>:"tm_getarea_a.vi"("error in (no error)"=w504, "Handle in"=w505) -> ("error out"=w528:errorcluster, "V Offset"=w530:T6, "H Offset"=w529:T6, "Handle out"=w527:u32, "H Width"=w531:T6, "V Width"=w532:T6)  [unwired: 4 in]
            n234 = Unbundle By Name(w529) -> ("Value"=w523:i32, "Minimum"=w526:i32, "Maximum"=w525:i32, "Increment"=w524:i32)
            n235 = Unbundle By Name(w530) -> ("Value"=w513:i32, "Minimum"=w522:i32, "Maximum"=w521:i32, "Increment"=w520:i32)
            n236 = Unbundle By Name(w531) -> ("Value"=w512:i32, "Minimum"=w519:i32, "Maximum"=w518:i32, "Increment"=w517:i32)
            n237 = Unbundle By Name(w532) -> ("Value"=w511:i32, "Minimum"=w516:i32, "Maximum"=w515:i32, "Increment"=w514:i32)
            n238 = property on="H Offset" class="DigNum (strict)"("Value"=w523, "Minimum"=w526, "Maximum"=w525, "Increment"=w524) -> ()  [unwired: 2 in, 2 out]
            n239 = property on="V Offset" class="DigNum (strict)"("Value"=w513, "Minimum"=w522, "Maximum"=w521, "Increment"=w520) -> ()  [unwired: 2 in, 2 out]
            n240 = property on="H Width" class="DigNum (strict)"("Value"=w512, "Minimum"=w519, "Maximum"=w518, "Increment"=w517) -> ()  [unwired: 2 in, 2 out]
            n241 = property on="V Width" class="DigNum (strict)"("Value"=w511, "Minimum"=w516, "Maximum"=w515, "Increment"=w514) -> ()  [unwired: 2 in, 2 out]
            n242 = local write "SHO"(w523) -> ()
            n243 = local write "SVO"(w513) -> ()
            n244 = local write "SHW"(w512) -> ()
            n245 = local write "SVW"(w511) -> ()
            n246 = call <userlib>:"tm_preparecapture.vi"("error in (no error)"=w528, "Capture mode"=w540, "Handle in"=w527) -> ("error out"=w538:errorcluster, "Buffer Info"=w535:T7, "Handle out"=w539:u32)  [unwired: 5 in, 1 out]
            n247 = call <userlib>:"tm_startcapture_b.vi"("error in (no error)"=w538, "Handle in"=w539) -> ("error out"=w537:errorcluster, "Handle out"=w536:u32)  [unwired: 8 in]
          }
          event "H Offset", "H Width", "V Offset", "V Width": Value Change {
            w585 = 1 items=["Snap", "Sequence"] ("Capture mode")
            n248 = event-data() -> ()  [unwired: 1 in, 4 out]
            n249 = call <userlib>:"tm_stopcapture.vi"("error in (no error)"=w547, "Handle in"=w548) -> ("error out"=w545:errorcluster, "Handle out"=w546:u32)  [unwired: 8 in]
            n250 = local read "H Offset"() -> (w551:i32)
            n251 = local read "H Width"() -> (w552:i32)
            n252 = local read "V Offset"() -> (w553:i32)
            n253 = local read "V Width"() -> (w550:i32)
            n254 = call <userlib>:"tm_unpreparecapture.vi"("error in (no error)"=w545, "Handle in"=w546) -> ("error out"=w543:errorcluster, "Handle out"=w544:u32)  [unwired: 8 in]
            n255 = Bundle("H Offset"=w551, "V Offset"=w553, "H Width"=w552, "V Width"=w550) -> (w549:T8)  [unwired: 1 in]
            n256 = call <userlib>:"tm_setarea.vi"("error in (no error)"=w543, "Sub Region"=w549, "Handle in"=w544) -> ("error out"=w554:errorcluster, "Handle out"=w555:u32)  [unwired: 7 in]
            n257 = call <userlib>:"tm_getarea_a.vi"("error in (no error)"=w554, "Handle in"=w555) -> ("error out"=w573:errorcluster, "V Offset"=w575:T6, "H Offset"=w574:T6, "Handle out"=w572:u32, "H Width"=w576:T6, "V Width"=w577:T6)  [unwired: 4 in]
            n258 = Unbundle By Name(w574) -> ("Value"=w568:i32, "Minimum"=w571:i32, "Maximum"=w570:i32, "Increment"=w569:i32)
            n259 = Unbundle By Name(w575) -> ("Value"=w558:i32, "Minimum"=w567:i32, "Maximum"=w566:i32, "Increment"=w565:i32)
            n260 = Unbundle By Name(w576) -> ("Value"=w557:i32, "Minimum"=w564:i32, "Maximum"=w563:i32, "Increment"=w562:i32)
            n261 = Unbundle By Name(w577) -> ("Value"=w556:i32, "Minimum"=w561:i32, "Maximum"=w560:i32, "Increment"=w559:i32)
            n262 = property on="H Offset" class="DigNum (strict)"("Value"=w568, "Minimum"=w571, "Maximum"=w570, "Increment"=w569) -> ()  [unwired: 2 in, 2 out]
            n263 = property on="V Offset" class="DigNum (strict)"("Value"=w558, "Minimum"=w567, "Maximum"=w566, "Increment"=w565) -> ()  [unwired: 2 in, 2 out]
            n264 = property on="H Width" class="DigNum (strict)"("Value"=w557, "Minimum"=w564, "Maximum"=w563, "Increment"=w562) -> ()  [unwired: 2 in, 2 out]
            n265 = property on="V Width" class="DigNum (strict)"("Value"=w556, "Minimum"=w561, "Maximum"=w560, "Increment"=w559) -> ()  [unwired: 2 in, 2 out]
            n266 = local write "SHO"(w568) -> ()
            n267 = local write "SVO"(w558) -> ()
            n268 = local write "SHW"(w557) -> ()
            n269 = local write "SVW"(w556) -> ()
            n270 = call <userlib>:"tm_preparecapture.vi"("error in (no error)"=w573, "Capture mode"=w585, "Handle in"=w572) -> ("error out"=w583:errorcluster, "Buffer Info"=w580:T7, "Handle out"=w584:u32)  [unwired: 5 in, 1 out]
            n271 = call <userlib>:"tm_startcapture_b.vi"("error in (no error)"=w583, "Handle in"=w584) -> ("error out"=w582:errorcluster, "Handle out"=w581:u32)  [unwired: 8 in]
          }
        }
        n272 = local read "stop"() -> (w89:bool)
        n273 = Unbundle By Name(w98) -> ("status"=w111:bool)
        n274 = Compound Arithmetic op=OR(w111, w89, w93) -> (w110:bool)
      }
      n275 = while {
        tunnel: w15 -> [w763]
        shift-right: [w759] -> _
        shift-left: _ -> [w757]
        shift-right: [w755] -> _
        shift-left: _ -> [w756]
        shift-right: [w753] -> _
        shift-left: _ -> [w749]
        stop <- w758 stop-if-true
        n276 = Dequeue Element(queue=w763) -> (element=w762:T2, timed out?=w750:bool)  [unwired: 2 in, 2 out]
        n277 = Unbundle By Name(w762) -> ("State"=w761:T1, "Stack Number"=w760:i32, "Image"=w751:u16[][])
        "State" <- w761
        n278 = case shown="False" w750 {
          tunnel: w751 -> [w765 w767]
          tunnel: [w765 w766] -> w752
          tunnel: [w764 w767] -> w753
          tunnel: w749 -> [w764 w766]
          frame False {
          }
          frame True {
          }
        }
        "Image" <- w752
        n279 = case shown="\"Idle\"" w761 {
          tunnel: w760 -> [_ _ _ _ _ _]
          tunnel: [w770 w787 _ _ _ _] -> w759
          tunnel: w757 -> [_ w788 w794 _ _ _]
          tunnel: [FALSE _ _ _ TRUE _] -> w758
          tunnel: w752 -> [w768 w789 _ _ _ _]
          tunnel: w756 -> [_ w786 w792 w804 w829 w831]
          tunnel: [w771 w785 w793 w800 w829 w831] -> w755
          tunnel: "Path" -> [w774 _ _ w806 _ _]
          frame "Start Sequence" {
            # "Public tiff library"
            # "Get path and open file"
            n280 = Equal?(x=w774, y=path "") -> (x = y?=w776:bool)
            n281 = case shown="True" w776 {
              tunnel: w774 -> [w778 _]
              tunnel: [w778 w781] -> w773
              frame False {
              }
              frame True {
                n282 = call "File Dialog"("pattern (all files)"=".tiff", "pattern label"="Tiff Image") -> ("selected path"=w781:path)  [unwired: 10 in, 3 out]
              }
            }
            n283 = case shown="False" "AutoIncrement" {
              tunnel: w773 -> [w782 w784]
              tunnel: [w782 w783] -> w769
              frame False {
              }
              frame True {
                n284 = call "4Digit File Incrementer.vi"("path"=w784) -> ("appended path"=w783:path)  [unwired: 10 in]
              }
            }
            n285 = call-poly "CTIFFNewFileAndStyle.vi"("image"=w768, "output_file"=w769) -> ("error"=w771:errorcluster, "CTIFF"=w770:i64)  [unwired: 8 in]
            n286 = local write "Path"(w769) -> ()
          }
          frame "Collecting" {
            # "Add Image to write scan line"
            n287 = call-poly "CTIFFAddNewPage.vi"("error"=w786, "image"=w789, "CTIFF"=w788) -> ("error"=w785:errorcluster, "CTIFF"=w787:i64)  [unwired: 7 in]
            n288 = property on="Ram Record" class="Bool (strict)"("DisabledEnum"=T4."Disabled and Grayed Out" ("Disabled"), "BoolText.Text"="Saving" ("Boolean Text.Text")) -> ()  [unwired: 2 in, 2 out]
          }
          frame "End" {
            (unwired) FALSE
            # "Close image file, reset capturing button"
            n289 = call "CTIFFWriteAndClose.vi"("error"=w792, "CTIFF"=w794) -> ("error"=w793:errorcluster)  [unwired: 9 in]
            n290 = property on="Ram Record" class="Bool (strict)"("BoolText.Text"="OK" ("Boolean Text.Text"), "DisabledEnum"=T4."Enabled" ("Disabled")) -> ()  [unwired: 2 in, 2 out]
          }
          frame "Read Disk" {
            n291 = local read "Temp"() -> (w801:path)
            n292 = call <userlib>:"tm_opendcimgfile.vi"("Path"=w801) -> ("Total Frames"=w807:i32, "File Handle"=w808:u32)  [unwired: 8 in, 1 out]
            n293 = for {
              N: w807 -> [_]
              tunnel: w806 -> [w816]
              shift-right: [w814] -> w802
              shift-left: i64 0 ("CTIFF") -> [w815]
              tunnel: [w813] -> w803
              tunnel: w804 -> [w812]
              shift-right: [w818] -> w797
              shift-left: w808 -> [w819]
              i -> [w810]
              n294 = Equal To 0?(x=w810) -> (x = 0?=w817:bool)
              n295 = call <userlib>:"tm_getdcimgframe.vi"("error in (no error)"=w812, "Frame Index"=w810, "File Handle in"=w819) -> ("error out"=w811:errorcluster, "Data"=w809:u16[][], "File Handle out"=w818:u32)  [unwired: 5 in, 1 out]
              n296 = local write "Image"(w809) -> ()
              n297 = case shown="True" w817 {
                tunnel: w816 -> [_ w828]
                tunnel: w809 -> [w820 w827]
                tunnel: w815 -> [w824 _]
                tunnel: [w823 w826] -> w814
                tunnel: [w822 w825] -> w813
                tunnel: w811 -> [w821 _]
                frame False {
                  n298 = call-poly "CTIFFAddNewPage.vi"("error"=w821, "image"=w820, "CTIFF"=w824) -> ("error"=w822:errorcluster, "CTIFF"=w823:i64)  [unwired: 7 in]
                }
                frame True {
                  n299 = call-poly "CTIFFNewFileAndStyle.vi"("image"=w827, "output_file"=w828) -> ("error"=w825:errorcluster, "CTIFF"=w826:i64)  [unwired: 8 in]
                }
              }
              "Frame Index" <- w810
            }
            n300 = call "CTIFFWriteAndClose.vi"("error"=w803, "CTIFF"=w802) -> ("error"=w799:errorcluster)  [unwired: 9 in]
            n301 = call <userlib>:"tm_closedcimgfile.vi"("error in (no error)"=w799, "File Handle"=w797) -> ("error out"=w798:errorcluster)  [unwired: 9 in]
            n302 = Delete(path (use dialog)=w801, error in=w798) -> (error out=w800:errorcluster)  [unwired: 3 in, 2 out]
          }
          frame "STOP" {
          }
          frame "Idle" {
          }
        }
      }
      n303 = call <userlib>:"tm_stopcapture.vi"("error in (no error)"=w9, "Handle in"=w10) -> ("error out"=w56:errorcluster, "Handle out"=w57:u32)  [unwired: 8 in]
      n304 = call <userlib>:"tm_unpreparecapture.vi"("error in (no error)"=w56, "Handle in"=w57) -> ("error out"=w55:errorcluster, "Handle out"=w58:u32)  [unwired: 8 in]
      n305 = call <userlib>:"tm_closecamera.vi"("error in (no error)"=w55, "Handle in"=w58) -> ("error out"=w85:errorcluster)  [unwired: 9 in]
      n306 = call <userlib>:"tm_deinitialize.vi"("error in (no error)"=w85) -> ("error out"=w84:errorcluster)  [unwired: 10 in]
    }
  }
  "error out" <- w3
